vi "Grid_multiGridV3.vi"() -> ()   [LabVIEW 2014]
panel:
  out "size(s) 5":i32
  out "size(s) 4":i32
  out "size(s) 3":i32=11
  out "size(s) 2":i32=12
  out "size(s)":i32=15
  out "data\n\n 5":T1(array[cluster])=[{"Amplitude (mod. signal unit)"=0.0, "Lockin on/off status"=FALSE, "Backward sweep"=TRUE, "Number of points"=215, "Channels"=["Current (A)", "LI Demod 1 X (A)", "LI Demod 1 Y (A)", "LI Demod 2 X (A)", "LI Demod 2 Y (A)"], "Parameters"=["X (m)", "Y (m)", "Z (m)", "Z offset (m)", "Settling time (s)", "Integration time (s)", "Z-Ctrl hold", "Final Z (m)"], "Fixed parameters"=["Sweep Start", "Sweep End"], "Multiple sweeps configuration"={"Number of Sweeps"=1, "Save all"=FALSE}, "Initialization"={"Z averaging time (s)"=0.001, "Initial settling time (s)"=0.0002}, "Sweep Timing"={"Max. slew rate (V/s)"=inf, "Settling time (s)"=0.001, "Integration time (s)"=0.001}, "End of Sweep"={"End settling time (s)"=5e-05, "Z control time (s)"=0.0002}, "Initial Z-Offset (m)"=0.0, "Sweep Distance (m)"=0.0, "Channels 2"=[], "Name"="", "Reset Z"=FALSE, "Record final Z"=FALSE, "Auto Retract Status"=FALSE, "Threshold"=0.0, "Auto Retract Signal Index"=0, "Auto Retract Condition"=FALSE}, {"Amplitude (mod. signal unit)"=0.0, "Lockin on/off status"=FALSE, "Backward sweep"=FALSE, "Number of points"=0, "Channels"=[], "Parameters"=[], "Fixed parameters"=[], "Multiple sweeps configuration"={"Number of Sweeps"=0, "Save all"=FALSE}, "Initialization"={"Z averaging time (s)"=0.0, "Initial settling time (s)"=0.0}, "Sweep Timing"={"Max. slew rate (V/s)"=0.0, "Settling time (s)"=0.0, "Integration time (s)"=0.0}, "End of Sweep"={"End settling time (s)"=0.0, "Z control time (s)"=0.0}, "Initial Z-Offset (m)"=0.0, "Sweep Distance (m)"=0.0, "Channels 2"=[], "Name"="", "Reset Z"=FALSE, "Record final Z"=FALSE, "Auto Retract Status"=FALSE, "Threshold"=0.0, "Auto Retract Signal Index"=0, "Auto Retract Condition"=FALSE}, {"Amplitude (mod. signal unit)"=0.0, "Lockin on/off status"=FALSE, "Backward sweep"=FALSE, "Number of points"=0, "Channels"=[], "Parameters"=[], "Fixed parameters"=[], "Multiple sweeps configuration"={"Number of Sweeps"=0, "Save all"=FALSE}, "Initialization"={"Z averaging time (s)"=0.0, "Initial settling time (s)"=0.0}, "Sweep Timing"={"Max. slew rate (V/s)"=0.0, "Settling time (s)"=0.0, "Integration time (s)"=0.0}, "End of Sweep"={"End settling time (s)"=0.0, "Z control time (s)"=0.0}, "Initial Z-Offset (m)"=0.0, "Sweep Distance (m)"=0.0, "Channels 2"=[], "Name"="", "Reset Z"=FALSE, "Record final Z"=FALSE, "Auto Retract Status"=FALSE, "Threshold"=0.0, "Auto Retract Signal Index"=0, "Auto Retract Condition"=FALSE}, {"Amplitude (mod. signal unit)"=0.0, "Lockin on/off status"=FALSE, "Backward sweep"=FALSE, "Number of points"=0, "Channels"=[], "Parameters"=[], "Fixed parameters"=[], "Multiple sweeps configuration"={"Number of Sweeps"=0, "Save all"=FALSE}, "Initialization"={"Z averaging time (s)"=0.0, "Initial settling time (s)"=0.0}, "Sweep Timing"={"Max. slew rate (V/s)"=0.0, "Settling time (s)"=0.0, "Integration time (s)"=0.0}, "End of Sweep"={"End settling time (s)"=0.0, "Z control time (s)"=0.0}, "Initial Z-Offset (m)"=0.0, "Sweep Distance (m)"=0.0, "Channels 2"=[], "Name"="", "Reset Z"=FALSE, "Record final Z"=FALSE, "Auto Retract Status"=FALSE, "Threshold"=0.0, "Auto Retract Signal Index"=0, "Auto Retract Condition"=FALSE}, {"Amplitude (mod. signal unit)"=0.0, "Lockin on/off status"=FALSE, "Backward sweep"=FALSE, "Number of points"=0, "Channels"=[], "Parameters"=[], "Fixed parameters"=[], "Multiple sweeps configuration"={"Number of Sweeps"=0, "Save all"=FALSE}, "Initialization"={"Z averaging time (s)"=0.0, "Initial settling time (s)"=0.0}, "Sweep Timing"={"Max. slew rate (V/s)"=0.0, "Settling time (s)"=0.0, "Integration time (s)"=0.0}, "End of Sweep"={"End settling time (s)"=0.0, "Z control time (s)"=0.0}, "Initial Z-Offset (m)"=0.0, "Sweep Distance (m)"=0.0, "Channels 2"=[], "Name"="", "Reset Z"=FALSE, "Record final Z"=FALSE, "Auto Retract Status"=FALSE, "Threshold"=0.0, "Auto Retract Signal Index"=0, "Auto Retract Condition"=FALSE}, {"Amplitude (mod. signal unit)"=0.0, "Lockin on/off status"=FALSE, "Backward sweep"=FALSE, "Number of points"=0, "Channels"=[], "Parameters"=[], "Fixed parameters"=[], "Multiple sweeps configuration"={"Number of Sweeps"=0, "Save all"=FALSE}, "Initialization"={"Z averaging time (s)"=0.0, "Initial settling time (s)"=0.0}, "Sweep Timing"={"Max. slew rate (V/s)"=0.0, "Settling time (s)"=0.0, "Integration time (s)"=0.0}, "End of Sweep"={"End settling time (s)"=0.0, "Z control time (s)"=0.0}, "Initial Z-Offset (m)"=0.0, "Sweep Distance (m)"=0.0, "Channels 2"=[], "Name"="", "Reset Z"=FALSE, "Record final Z"=FALSE, "Auto Retract Status"=FALSE, "Threshold"=0.0, "Auto Retract Signal Index"=0, "Auto Retract Condition"=FALSE}, {"Amplitude (mod. signal unit)"=0.0, "Lockin on/off status"=FALSE, "Backward sweep"=FALSE, "Number of points"=0, "Channels"=[], "Parameters"=[], "Fixed parameters"=[], "Multiple sweeps configuration"={"Number of Sweeps"=0, "Save all"=FALSE}, "Initialization"={"Z averaging time (s)"=0.0, "Initial settling time (s)"=0.0}, "Sweep Timing"={"Max. slew rate (V/s)"=0.0, "Settling time (s)"=0.0, "Integration time (s)"=0.0}, "End of Sweep"={"End settling time (s)"=0.0, "Z control time (s)"=0.0}, "Initial Z-Offset (m)"=0.0, "Sweep Distance (m)"=0.0, "Channels 2"=[], "Name"="", "Reset Z"=FALSE, "Record final Z"=FALSE, "Auto Retract Status"=FALSE, "Threshold"=0.0, "Auto Retract Signal Index"=0, "Auto Retract Condition"=FALSE}, {"Amplitude (mod. signal unit)"=0.0, "Lockin on/off status"=FALSE, "Backward sweep"=FALSE, "Number of points"=0, "Channels"=[], "Parameters"=[], "Fixed parameters"=[], "Multiple sweeps configuration"={"Number of Sweeps"=0, "Save all"=FALSE}, "Initialization"={"Z averaging time (s)"=0.0, "Initial settling time (s)"=0.0}, "Sweep Timing"={"Max. slew rate (V/s)"=0.0, "Settling time (s)"=0.0, "Integration time (s)"=0.0}, "End of Sweep"={"End settling time (s)"=0.0, "Z control time (s)"=0.0}, "Initial Z-Offset (m)"=0.0, "Sweep Distance (m)"=0.0, "Channels 2"=[], "Name"="", "Reset Z"=FALSE, "Record final Z"=FALSE, "Auto Retract Status"=FALSE, "Threshold"=0.0, "Auto Retract Signal Index"=0, "Auto Retract Condition"=FALSE}, {"Amplitude (mod. signal unit)"=0.0, "Lockin on/off status"=FALSE, "Backward sweep"=FALSE, "Number of points"=0, "Channels"=[], "Parameters"=[], "Fixed parameters"=[], "Multiple sweeps configuration"={"Number of Sweeps"=0, "Save all"=FALSE}, "Initialization"={"Z averaging time (s)"=0.0, "Initial settling time (s)"=0.0}, "Sweep Timing"={"Max. slew rate (V/s)"=0.0, "Settling time (s)"=0.0, "Integration time (s)"=0.0}, "End of Sweep"={"End settling time (s)"=0.0, "Z control time (s)"=0.0}, "Initial Z-Offset (m)"=0.0, "Sweep Distance (m)"=0.0, "Channels 2"=[], "Name"="", "Reset Z"=FALSE, "Record final Z"=FALSE, "Auto Retract Status"=FALSE, "Threshold"=0.0, "Auto Retract Signal Index"=0, "Auto Retract Condition"=FALSE}, {"Amplitude (mod. signal unit)"=0.0, "Lockin on/off status"=FALSE, "Backward sweep"=FALSE, "Number of points"=0, "Channels"=[], "Parameters"=[], "Fixed parameters"=[], "Multiple sweeps configuration"={"Number of Sweeps"=0, "Save all"=FALSE}, "Initialization"={"Z averaging time (s)"=0.0, "Initial settling time (s)"=0.0}, "Sweep Timing"={"Max. slew rate (V/s)"=0.0, "Settling time (s)"=0.0, "Integration time (s)"=0.0}, "End of Sweep"={"End settling time (s)"=0.0, "Z control time (s)"=0.0}, "Initial Z-Offset (m)"=0.0, "Sweep Distance (m)"=0.0, "Channels 2"=[], "Name"="", "Reset Z"=FALSE, "Record final Z"=FALSE, "Auto Retract Status"=FALSE, "Threshold"=0.0, "Auto Retract Signal Index"=0, "Auto Retract Condition"=FALSE}, {"Amplitude (mod. signal unit)"=0.0, "Lockin on/off status"=FALSE, "Backward sweep"=FALSE, "Number of points"=0, "Channels"=[], "Parameters"=[], "Fixed parameters"=[], "Multiple sweeps configuration"={"Number of Sweeps"=0, "Save all"=FALSE}, "Initialization"={"Z averaging time (s)"=0.0, "Initial settling time (s)"=0.0}, "Sweep Timing"={"Max. slew rate (V/s)"=0.0, "Settling time (s)"=0.0, "Integration time (s)"=0.0}, "End of Sweep"={"End settling time (s)"=0.0, "Z control time (s)"=0.0}, "Initial Z-Offset (m)"=0.0, "Sweep Distance (m)"=0.0, "Channels 2"=[], "Name"="", "Reset Z"=FALSE, "Record final Z"=FALSE, "Auto Retract Status"=FALSE, "Threshold"=0.0, "Auto Retract Signal Index"=0, "Auto Retract Condition"=FALSE}, {"Amplitude (mod. signal unit)"=0.0, "Lockin on/off status"=FALSE, "Backward sweep"=FALSE, "Number of points"=0, "Channels"=[], "Parameters"=[], "Fixed parameters"=[], "Multiple sweeps configuration"={"Number of Sweeps"=0, "Save all"=FALSE}, "Initialization"={"Z averaging time (s)"=0.0, "Initial settling time (s)"=0.0}, "Sweep Timing"={"Max. slew rate (V/s)"=0.0, "Settling time (s)"=0.0, "Integration time (s)"=0.0}, "End of Sweep"={"End settling time (s)"=0.0, "Z control time (s)"=0.0}, "Initial Z-Offset (m)"=0.0, "Sweep Distance (m)"=0.0, "Channels 2"=[], "Name"="", "Reset Z"=FALSE, "Record final Z"=FALSE, "Auto Retract Status"=FALSE, "Threshold"=0.0, "Auto Retract Signal Index"=0, "Auto Retract Condition"=FALSE}, {"Amplitude (mod. signal unit)"=0.0, "Lockin on/off status"=FALSE, "Backward sweep"=FALSE, "Number of points"=0, "Channels"=[], "Parameters"=[], "Fixed parameters"=[], "Multiple sweeps configuration"={"Number of Sweeps"=0, "Save all"=FALSE}, "Initialization"={"Z averaging time (s)"=0.0, "Initial settling time (s)"=0.0}, "Sweep Timing"={"Max. slew rate (V/s)"=0.0, "Settling time (s)"=0.0, "Integration time (s)"=0.0}, "End of Sweep"={"End settling time (s)"=0.0, "Z control time (s)"=0.0}, "Initial Z-Offset (m)"=0.0, "Sweep Distance (m)"=0.0, "Channels 2"=[], "Name"="", "Reset Z"=FALSE, "Record final Z"=FALSE, "Auto Retract Status"=FALSE, "Threshold"=0.0, "Auto Retract Signal Index"=0, "Auto Retract Condition"=FALSE}, {"Amplitude (mod. signal unit)"=0.0, "Lockin on/off status"=FALSE, "Backward sweep"=FALSE, "Number of points"=0, "Channels"=[], "Parameters"=[], "Fixed parameters"=[], "Multiple sweeps configuration"={"Number of Sweeps"=0, "Save all"=FALSE}, "Initialization"={"Z averaging time (s)"=0.0, "Initial settling time (s)"=0.0}, "Sweep Timing"={"Max. slew rate (V/s)"=0.0, "Settling time (s)"=0.0, "Integration time (s)"=0.0}, "End of Sweep"={"End settling time (s)"=0.0, "Z control time (s)"=0.0}, "Initial Z-Offset (m)"=0.0, "Sweep Distance (m)"=0.0, "Channels 2"=[], "Name"="", "Reset Z"=FALSE, "Record final Z"=FALSE, "Auto Retract Status"=FALSE, "Threshold"=0.0, "Auto Retract Signal Index"=0, "Auto Retract Condition"=FALSE}, {"Amplitude (mod. signal unit)"=0.0, "Lockin on/off status"=FALSE, "Backward sweep"=FALSE, "Number of points"=0, "Channels"=[], "Parameters"=[], "Fixed parameters"=[], "Multiple sweeps configuration"={"Number of Sweeps"=0, "Save all"=FALSE}, "Initialization"={"Z averaging time (s)"=0.0, "Initial settling time (s)"=0.0}, "Sweep Timing"={"Max. slew rate (V/s)"=0.0, "Settling time (s)"=0.0, "Integration time (s)"=0.0}, "End of Sweep"={"End settling time (s)"=0.0, "Z control time (s)"=0.0}, "Initial Z-Offset (m)"=0.0, "Sweep Distance (m)"=0.0, "Channels 2"=[], "Name"="", "Reset Z"=FALSE, "Record final Z"=FALSE, "Auto Retract Status"=FALSE, "Threshold"=0.0, "Auto Retract Signal Index"=0, "Auto Retract Condition"=FALSE}, {"Amplitude (mod. signal unit)"=0.0, "Lockin on/off status"=FALSE, "Backward sweep"=FALSE, "Number of points"=0, "Channels"=[], "Parameters"=[], "Fixed parameters"=[], "Multiple sweeps configuration"={"Number of Sweeps"=0, "Save all"=FALSE}, "Initialization"={"Z averaging time (s)"=0.0, "Initial settling time (s)"=0.0}, "Sweep Timing"={"Max. slew rate (V/s)"=0.0, "Settling time (s)"=0.0, "Integration time (s)"=0.0}, "End of Sweep"={"End settling time (s)"=0.0, "Z control time (s)"=0.0}, "Initial Z-Offset (m)"=0.0, "Sweep Distance (m)"=0.0, "Channels 2"=[], "Name"="", "Reset Z"=FALSE, "Record final Z"=FALSE, "Auto Retract Status"=FALSE, "Threshold"=0.0, "Auto Retract Signal Index"=0, "Auto Retract Condition"=FALSE}, {"Amplitude (mod. signal unit)"=0.0, "Lockin on/off status"=FALSE, "Backward sweep"=FALSE, "Number of points"=0, "Channels"=[], "Parameters"=[], "Fixed parameters"=[], "Multiple sweeps configuration"={"Number of Sweeps"=0, "Save all"=FALSE}, "Initialization"={"Z averaging time (s)"=0.0, "Initial settling time (s)"=0.0}, "Sweep Timing"={"Max. slew rate (V/s)"=0.0, "Settling time (s)"=0.0, "Integration time (s)"=0.0}, "End of Sweep"={"End settling time (s)"=0.0, "Z control time (s)"=0.0}, "Initial Z-Offset (m)"=0.0, "Sweep Distance (m)"=0.0, "Channels 2"=[], "Name"="", "Reset Z"=FALSE, "Record final Z"=FALSE, "Auto Retract Status"=FALSE, "Threshold"=0.0, "Auto Retract Signal Index"=0, "Auto Retract Condition"=FALSE}, {"Amplitude (mod. signal unit)"=0.0, "Lockin on/off status"=FALSE, "Backward sweep"=FALSE, "Number of points"=0, "Channels"=[], "Parameters"=[], "Fixed parameters"=[], "Multiple sweeps configuration"={"Number of Sweeps"=0, "Save all"=FALSE}, "Initialization"={"Z averaging time (s)"=0.0, "Initial settling time (s)"=0.0}, "Sweep Timing"={"Max. slew rate (V/s)"=0.0, "Settling time (s)"=0.0, "Integration time (s)"=0.0}, "End of Sweep"={"End settling time (s)"=0.0, "Z control time (s)"=0.0}, "Initial Z-Offset (m)"=0.0, "Sweep Distance (m)"=0.0, "Channels 2"=[], "Name"="", "Reset Z"=FALSE, "Record final Z"=FALSE, "Auto Retract Status"=FALSE, "Threshold"=0.0, "Auto Retract Signal Index"=0, "Auto Retract Condition"=FALSE}]
  out "data\n\n 2":T2(array[cluster])=[{"Amplitude (mod. signal unit)"=0.0, "Lockin on/off status"=FALSE, "Advanced options"={"Z-Controller Hold"=TRUE, "Record final Z"=FALSE, "Reset Bias"=TRUE}, "Backward sweep"=TRUE, "Number of points"=215, "Channels"=["Current (A)", "LI Demod 1 X (A)", "LI Demod 1 Y (A)", "LI Demod 2 X (A)", "LI Demod 2 Y (A)"], "Parameters"=["X (m)", "Y (m)", "Z (m)", "Z offset (m)", "Settling time (s)", "Integration time (s)", "Z-Ctrl hold", "Final Z (m)"], "Fixed parameters"=["Sweep Start", "Sweep End"], "Multiple sweeps configuration"={"Number of Sweeps"=1, "Save all"=FALSE}, "Initialization"={"Z averaging time (s)"=0.001, "Z offset (m)"=0.0, "Initial settling time (s)"=0.0002}, "Sweep Timing"={"Max. slew rate (V/s)"=inf, "Settling time (s)"=0.001, "Integration time (s)"=0.001}, "End of Sweep"={"End settling time (s)"=5e-05, "Z control time (s)"=0.0002}, "Start value (V)"=-0.02, "End value (V)"=-3.0, "Channels 2"=[0, 20, 21, 22, 23], "Name"="numerical_DCA_-20mV->-3V"}, {"Amplitude (mod. signal unit)"=0.0, "Lockin on/off status"=FALSE, "Advanced options"={"Z-Controller Hold"=TRUE, "Record final Z"=FALSE, "Reset Bias"=TRUE}, "Backward sweep"=TRUE, "Number of points"=215, "Channels"=["Current (A)", "LI Demod 1 X (A)", "LI Demod 1 Y (A)", "LI Demod 2 X (A)", "LI Demod 2 Y (A)"], "Parameters"=["X (m)", "Y (m)", "Z (m)", "Z offset (m)", "Settling time (s)", "Integration time (s)", "Z-Ctrl hold", "Final Z (m)"], "Fixed parameters"=["Sweep Start", "Sweep End"], "Multiple sweeps configuration"={"Number of Sweeps"=1, "Save all"=FALSE}, "Initialization"={"Z averaging time (s)"=0.001, "Z offset (m)"=0.0, "Initial settling time (s)"=0.0002}, "Sweep Timing"={"Max. slew rate (V/s)"=inf, "Settling time (s)"=0.001, "Integration time (s)"=0.001}, "End of Sweep"={"End settling time (s)"=5e-05, "Z control time (s)"=0.0002}, "Start value (V)"=-0.02, "End value (V)"=0.7, "Channels 2"=[0, 20, 21, 22, 23], "Name"="numerical_DCA_-20mV->0.7V"}, {"Amplitude (mod. signal unit)"=0.0, "Lockin on/off status"=FALSE, "Advanced options"={"Z-Controller Hold"=TRUE, "Record final Z"=FALSE, "Reset Bias"=TRUE}, "Backward sweep"=TRUE, "Number of points"=215, "Channels"=["Current (A)", "LI Demod 1 X (A)", "LI Demod 1 Y (A)", "LI Demod 2 X (A)", "LI Demod 2 Y (A)"], "Parameters"=["X (m)", "Y (m)", "Z (m)", "Z offset (m)", "Settling time (s)", "Integration time (s)", "Z-Ctrl hold", "Final Z (m)"], "Fixed parameters"=["Sweep Start", "Sweep End"], "Multiple sweeps configuration"={"Number of Sweeps"=30, "Save all"=FALSE}, "Initialization"={"Z averaging time (s)"=0.001, "Z offset (m)"=0.0, "Initial settling time (s)"=0.0002}, "Sweep Timing"={"Max. slew rate (V/s)"=inf, "Settling time (s)"=0.001, "Integration time (s)"=0.001}, "End of Sweep"={"End settling time (s)"=5e-05, "Z control time (s)"=0.0002}, "Start value (V)"=-0.02, "End value (V)"=0.7, "Channels 2"=[0, 20, 21, 22, 23], "Name"="numerical_DCA_-20mV->-0.7V_30sweeps"}, {"Amplitude (mod. signal unit)"=0.0, "Lockin on/off status"=FALSE, "Advanced options"={"Z-Controller Hold"=TRUE, "Record final Z"=FALSE, "Reset Bias"=TRUE}, "Backward sweep"=TRUE, "Number of points"=215, "Channels"=["Current (A)", "LI Demod 1 X (A)", "LI Demod 1 Y (A)", "LI Demod 2 X (A)", "LI Demod 2 Y (A)"], "Parameters"=["X (m)", "Y (m)", "Z (m)", "Z offset (m)", "Settling time (s)", "Integration time (s)", "Z-Ctrl hold", "Final Z (m)"], "Fixed parameters"=["Sweep Start", "Sweep End"], "Multiple sweeps configuration"={"Number of Sweeps"=50, "Save all"=FALSE}, "Initialization"={"Z averaging time (s)"=0.001, "Z offset (m)"=0.0, "Initial settling time (s)"=0.0002}, "Sweep Timing"={"Max. slew rate (V/s)"=inf, "Settling time (s)"=0.001, "Integration time (s)"=0.001}, "End of Sweep"={"End settling time (s)"=5e-05, "Z control time (s)"=0.0002}, "Start value (V)"=-0.02, "End value (V)"=0.7, "Channels 2"=[0, 20, 21, 22, 23], "Name"="numerical_DCA_-20mV->-0.7V_50_sweeps"}, {"Amplitude (mod. signal unit)"=0.0, "Lockin on/off status"=FALSE, "Advanced options"={"Z-Controller Hold"=TRUE, "Record final Z"=FALSE, "Reset Bias"=TRUE}, "Backward sweep"=TRUE, "Number of points"=215, "Channels"=["Current (A)", "LI Demod 1 X (A)", "LI Demod 1 Y (A)", "LI Demod 2 X (A)", "LI Demod 2 Y (A)"], "Parameters"=["X (m)", "Y (m)", "Z (m)", "Z offset (m)", "Settling time (s)", "Integration time (s)", "Z-Ctrl hold", "Final Z (m)"], "Fixed parameters"=["Sweep Start", "Sweep End"], "Multiple sweeps configuration"={"Number of Sweeps"=70, "Save all"=FALSE}, "Initialization"={"Z averaging time (s)"=0.001, "Z offset (m)"=0.0, "Initial settling time (s)"=0.0002}, "Sweep Timing"={"Max. slew rate (V/s)"=inf, "Settling time (s)"=0.001, "Integration time (s)"=0.001}, "End of Sweep"={"End settling time (s)"=5e-05, "Z control time (s)"=0.0002}, "Start value (V)"=-0.02, "End value (V)"=-3.0, "Channels 2"=[0, 20, 21, 22, 23], "Name"="numerical_DCA_-20mV->-3V_70sweeps"}, {"Amplitude (mod. signal unit)"=0.0, "Lockin on/off status"=FALSE, "Advanced options"={"Z-Controller Hold"=TRUE, "Record final Z"=FALSE, "Reset Bias"=TRUE}, "Backward sweep"=TRUE, "Number of points"=215, "Channels"=["Current (A)", "LI Demod 1 X (A)", "LI Demod 1 Y (A)", "LI Demod 2 X (A)", "LI Demod 2 Y (A)"], "Parameters"=["X (m)", "Y (m)", "Z (m)", "Z offset (m)", "Settling time (s)", "Integration time (s)", "Z-Ctrl hold", "Final Z (m)"], "Fixed parameters"=["Sweep Start", "Sweep End"], "Multiple sweeps configuration"={"Number of Sweeps"=100, "Save all"=FALSE}, "Initialization"={"Z averaging time (s)"=0.001, "Z offset (m)"=0.0, "Initial settling time (s)"=0.0002}, "Sweep Timing"={"Max. slew rate (V/s)"=inf, "Settling time (s)"=0.001, "Integration time (s)"=0.001}, "End of Sweep"={"End settling time (s)"=5e-05, "Z control time (s)"=0.0002}, "Start value (V)"=-0.02, "End value (V)"=-3.0, "Channels 2"=[0, 20, 21, 22, 23], "Name"="numerical_DCA_-20mV->3V_100_sweeps"}, {"Amplitude (mod. signal unit)"=0.0, "Lockin on/off status"=FALSE, "Advanced options"={"Z-Controller Hold"=TRUE, "Record final Z"=FALSE, "Reset Bias"=TRUE}, "Backward sweep"=TRUE, "Number of points"=256, "Channels"=["Current (A)", "LI Demod 1 X (A)", "LI Demod 1 Y (A)", "LI Demod 2 X (A)", "LI Demod 2 Y (A)"], "Parameters"=["X (m)", "Y (m)", "Z (m)", "Z offset (m)", "Settling time (s)", "Integration time (s)", "Z-Ctrl hold", "Final Z (m)"], "Fixed parameters"=["Sweep Start", "Sweep End"], "Multiple sweeps configuration"={"Number of Sweeps"=100, "Save all"=FALSE}, "Initialization"={"Z averaging time (s)"=0.001, "Z offset (m)"=0.0, "Initial settling time (s)"=5e-05}, "Sweep Timing"={"Max. slew rate (V/s)"=inf, "Settling time (s)"=0.001, "Integration time (s)"=0.0005}, "End of Sweep"={"End settling time (s)"=5e-05, "Z control time (s)"=5e-05}, "Start value (V)"=-1.0, "End value (V)"=2.0, "Channels 2"=[0, 20, 21, 22, 23], "Name"="numerical_-1V->2V"}, {"Amplitude (mod. signal unit)"=0.0, "Lockin on/off status"=FALSE, "Advanced options"={"Z-Controller Hold"=TRUE, "Record final Z"=FALSE, "Reset Bias"=TRUE}, "Backward sweep"=TRUE, "Number of points"=256, "Channels"=["Current (A)", "LI Demod 1 X (A)", "LI Demod 1 Y (A)", "LI Demod 2 X (A)", "LI Demod 2 Y (A)"], "Parameters"=["X (m)", "Y (m)", "Z (m)", "Z offset (m)", "Settling time (s)", "Integration time (s)", "Z-Ctrl hold", "Final Z (m)"], "Fixed parameters"=["Sweep Start", "Sweep End"], "Multiple sweeps configuration"={"Number of Sweeps"=100, "Save all"=FALSE}, "Initialization"={"Z averaging time (s)"=0.001, "Z offset (m)"=0.0, "Initial settling time (s)"=5e-05}, "Sweep Timing"={"Max. slew rate (V/s)"=inf, "Settling time (s)"=0.001, "Integration time (s)"=0.0005}, "End of Sweep"={"End settling time (s)"=5e-05, "Z control time (s)"=5e-05}, "Start value (V)"=-0.02, "End value (V)"=0.02, "Channels 2"=[0, 20, 21, 22, 23], "Name"="numerical_-20mV->20mV"}, {"Amplitude (mod. signal unit)"=0.0, "Lockin on/off status"=FALSE, "Advanced options"={"Z-Controller Hold"=TRUE, "Record final Z"=FALSE, "Reset Bias"=TRUE}, "Backward sweep"=TRUE, "Number of points"=286, "Channels"=["Current (A)", "LI Demod 1 X (A)", "LI Demod 1 Y (A)", "LI Demod 2 X (A)", "LI Demod 2 Y (A)"], "Parameters"=["X (m)", "Y (m)", "Z (m)", "Z offset (m)", "Settling time (s)", "Integration time (s)", "Z-Ctrl hold", "Final Z (m)"], "Fixed parameters"=["Sweep Start", "Sweep End"], "Multiple sweeps configuration"={"Number of Sweeps"=50, "Save all"=FALSE}, "Initialization"={"Z averaging time (s)"=0.001, "Z offset (m)"=0.0, "Initial settling time (s)"=5e-05}, "Sweep Timing"={"Max. slew rate (V/s)"=inf, "Settling time (s)"=0.001, "Integration time (s)"=0.0005}, "End of Sweep"={"End settling time (s)"=5e-05, "Z control time (s)"=5e-05}, "Start value (V)"=-0.2, "End value (V)"=0.8, "Channels 2"=[0, 20, 21, 22, 23], "Name"="DCA_numerical_-0.2V->0.8V"}, {"Amplitude (mod. signal unit)"=0.0, "Lockin on/off status"=FALSE, "Advanced options"={"Z-Controller Hold"=TRUE, "Record final Z"=FALSE, "Reset Bias"=TRUE}, "Backward sweep"=TRUE, "Number of points"=421, "Channels"=["Current (A)", "LI Demod 1 X (A)", "LI Demod 1 Y (A)", "LI Demod 2 X (A)", "LI Demod 2 Y (A)"], "Parameters"=["X (m)", "Y (m)", "Z (m)", "Z offset (m)", "Settling time (s)", "Integration time (s)", "Z-Ctrl hold", "Final Z (m)"], "Fixed parameters"=["Sweep Start", "Sweep End"], "Multiple sweeps configuration"={"Number of Sweeps"=100, "Save all"=FALSE}, "Initialization"={"Z averaging time (s)"=0.001, "Z offset (m)"=0.0, "Initial settling time (s)"=5e-05}, "Sweep Timing"={"Max. slew rate (V/s)"=inf, "Settling time (s)"=0.001, "Integration time (s)"=0.0005}, "End of Sweep"={"End settling time (s)"=5e-05, "Z control time (s)"=5e-05}, "Start value (V)"=-2.0, "End value (V)"=2.2, "Channels 2"=[0, 20, 21, 22, 23], "Name"="numerical_-2V->2.2V"}, {"Amplitude (mod. signal unit)"=0.0, "Lockin on/off status"=FALSE, "Advanced options"={"Z-Controller Hold"=TRUE, "Record final Z"=FALSE, "Reset Bias"=TRUE}, "Backward sweep"=TRUE, "Number of points"=500, "Channels"=["Current (A)", "LI Demod 1 X (A)", "LI Demod 1 Y (A)", "LI Demod 2 X (A)", "LI Demod 2 Y (A)"], "Parameters"=["X (m)", "Y (m)", "Z (m)", "Z offset (m)", "Settling time (s)", "Integration time (s)", "Z-Ctrl hold", "Final Z (m)"], "Fixed parameters"=["Sweep Start", "Sweep End"], "Multiple sweeps configuration"={"Number of Sweeps"=20, "Save all"=FALSE}, "Initialization"={"Z averaging time (s)"=0.001, "Z offset (m)"=0.0, "Initial settling time (s)"=0.01}, "Sweep Timing"={"Max. slew rate (V/s)"=inf, "Settling time (s)"=0.001, "Integration time (s)"=0.001}, "End of Sweep"={"End settling time (s)"=0.1, "Z control time (s)"=0.001}, "Start value (V)"=-0.2, "End value (V)"=0.8, "Channels 2"=[0, 20, 21, 22, 23], "Name"="DCA_numerical2_-0.2V->0.8V"}, {"Amplitude (mod. signal unit)"=0.0015, "Lockin on/off status"=FALSE, "Advanced options"={"Z-Controller Hold"=TRUE, "Record final Z"=FALSE, "Reset Bias"=TRUE}, "Backward sweep"=TRUE, "Number of points"=80, "Channels"=["Current (A)", "LI Demod 1 X (A)", "LI Demod 1 Y (A)", "LI Demod 2 X (A)", "LI Demod 2 Y (A)"], "Parameters"=["X (m)", "Y (m)", "Z (m)", "Z offset (m)", "Settling time (s)", "Integration time (s)", "Z-Ctrl hold", "Final Z (m)"], "Fixed parameters"=["Sweep Start", "Sweep End"], "Multiple sweeps configuration"={"Number of Sweeps"=10, "Save all"=FALSE}, "Initialization"={"Z averaging time (s)"=0.001, "Z offset (m)"=0.0, "Initial settling time (s)"=0.0046}, "Sweep Timing"={"Max. slew rate (V/s)"=inf, "Settling time (s)"=0.0046, "Integration time (s)"=0.032}, "End of Sweep"={"End settling time (s)"=5e-05, "Z control time (s)"=5e-05}, "Start value (V)"=-0.02, "End value (V)"=0.02, "Channels 2"=[0, 20, 21, 22, 23], "Name"="lockin_-20mV->20mV"}, {"Amplitude (mod. signal unit)"=0.002, "Lockin on/off status"=FALSE, "Advanced options"={"Z-Controller Hold"=TRUE, "Record final Z"=FALSE, "Reset Bias"=TRUE}, "Backward sweep"=TRUE, "Number of points"=70, "Channels"=["Current (A)", "LI Demod 1 X (A)", "LI Demod 1 Y (A)", "LI Demod 2 X (A)", "LI Demod 2 Y (A)"], "Parameters"=["X (m)", "Y (m)", "Z (m)", "Z offset (m)", "Settling time (s)", "Integration time (s)", "Z-Ctrl hold", "Final Z (m)"], "Fixed parameters"=["Sweep Start", "Sweep End"], "Multiple sweeps configuration"={"Number of Sweeps"=10, "Save all"=FALSE}, "Initialization"={"Z averaging time (s)"=0.001, "Z offset (m)"=0.0, "Initial settling time (s)"=0.0046}, "Sweep Timing"={"Max. slew rate (V/s)"=inf, "Settling time (s)"=0.0046, "Integration time (s)"=0.032}, "End of Sweep"={"End settling time (s)"=5e-05, "Z control time (s)"=5e-05}, "Start value (V)"=-0.025, "End value (V)"=0.025, "Channels 2"=[0, 20, 21, 22, 23], "Name"="lockin_-25mV->25mV"}, {"Amplitude (mod. signal unit)"=0.002, "Lockin on/off status"=FALSE, "Advanced options"={"Z-Controller Hold"=TRUE, "Record final Z"=FALSE, "Reset Bias"=TRUE}, "Backward sweep"=TRUE, "Number of points"=70, "Channels"=["Current (A)", "LI Demod 1 X (A)", "LI Demod 1 Y (A)", "LI Demod 2 X (A)", "LI Demod 2 Y (A)"], "Parameters"=["X (m)", "Y (m)", "Z (m)", "Z offset (m)", "Settling time (s)", "Integration time (s)", "Z-Ctrl hold", "Final Z (m)"], "Fixed parameters"=["Sweep Start", "Sweep End"], "Multiple sweeps configuration"={"Number of Sweeps"=10, "Save all"=FALSE}, "Initialization"={"Z averaging time (s)"=0.001, "Z offset (m)"=0.0, "Initial settling time (s)"=0.0046}, "Sweep Timing"={"Max. slew rate (V/s)"=inf, "Settling time (s)"=0.0046, "Integration time (s)"=0.032}, "End of Sweep"={"End settling time (s)"=5e-05, "Z control time (s)"=5e-05}, "Start value (V)"=-0.025, "End value (V)"=0.025, "Channels 2"=[0, 20, 21, 22, 23], "Name"="test"}, {"Amplitude (mod. signal unit)"=0.0025, "Lockin on/off status"=FALSE, "Advanced options"={"Z-Controller Hold"=TRUE, "Record final Z"=FALSE, "Reset Bias"=TRUE}, "Backward sweep"=TRUE, "Number of points"=320, "Channels"=["Current (A)", "LI Demod 1 X (A)", "LI Demod 1 Y (A)", "LI Demod 2 X (A)", "LI Demod 2 Y (A)"], "Parameters"=["X (m)", "Y (m)", "Z (m)", "Z offset (m)", "Settling time (s)", "Integration time (s)", "Z-Ctrl hold", "Final Z (m)"], "Fixed parameters"=["Sweep Start", "Sweep End"], "Multiple sweeps configuration"={"Number of Sweeps"=1, "Save all"=FALSE}, "Initialization"={"Z averaging time (s)"=0.001, "Z offset (m)"=0.0, "Initial settling time (s)"=0.0046}, "Sweep Timing"={"Max. slew rate (V/s)"=inf, "Settling time (s)"=0.0046, "Integration time (s)"=0.0042}, "End of Sweep"={"End settling time (s)"=5e-05, "Z control time (s)"=5e-05}, "Start value (V)"=0.02, "End value (V)"=-0.02, "Channels 2"=[0, 20, 21, 22, 23], "Name"="lockin_highRes_20mV_-20mV"}, {"Amplitude (mod. signal unit)"=0.005, "Lockin on/off status"=FALSE, "Advanced options"={"Z-Controller Hold"=TRUE, "Record final Z"=FALSE, "Reset Bias"=TRUE}, "Backward sweep"=TRUE, "Number of points"=256, "Channels"=["Current (A)", "LI Demod 1 X (A)", "LI Demod 1 Y (A)", "LI Demod 2 X (A)", "LI Demod 2 Y (A)"], "Parameters"=["X (m)", "Y (m)", "Z (m)", "Z offset (m)", "Settling time (s)", "Integration time (s)", "Z-Ctrl hold", "Final Z (m)"], "Fixed parameters"=["Sweep Start", "Sweep End"], "Multiple sweeps configuration"={"Number of Sweeps"=2, "Save all"=FALSE}, "Initialization"={"Z averaging time (s)"=0.001, "Z offset (m)"=0.0, "Initial settling time (s)"=0.0033}, "Sweep Timing"={"Max. slew rate (V/s)"=inf, "Settling time (s)"=0.0033, "Integration time (s)"=0.0164}, "End of Sweep"={"End settling time (s)"=5e-05, "Z control time (s)"=5e-05}, "Start value (V)"=-1.0, "End value (V)"=2.0, "Channels 2"=[0, 20, 21, 22, 23], "Name"="lockin_slow"}, {"Amplitude (mod. signal unit)"=0.005, "Lockin on/off status"=FALSE, "Advanced options"={"Z-Controller Hold"=TRUE, "Record final Z"=FALSE, "Reset Bias"=TRUE}, "Backward sweep"=TRUE, "Number of points"=310, "Channels"=["Current (A)", "LI Demod 1 X (A)", "LI Demod 1 Y (A)", "LI Demod 2 X (A)", "LI Demod 2 Y (A)"], "Parameters"=["X (m)", "Y (m)", "Z (m)", "Z offset (m)", "Settling time (s)", "Integration time (s)", "Z-Ctrl hold", "Final Z (m)"], "Fixed parameters"=["Sweep Start", "Sweep End"], "Multiple sweeps configuration"={"Number of Sweeps"=2, "Save all"=FALSE}, "Initialization"={"Z averaging time (s)"=0.001, "Z offset (m)"=0.0, "Initial settling time (s)"=0.0031}, "Sweep Timing"={"Max. slew rate (V/s)"=inf, "Settling time (s)"=0.0031, "Integration time (s)"=0.0246}, "End of Sweep"={"End settling time (s)"=5e-05, "Z control time (s)"=5e-05}, "Start value (V)"=1.5, "End value (V)"=-0.05, "Channels 2"=[0, 20, 21, 22, 23], "Name"="Lock_in_DCA_1.5V->-50mV"}, {"Amplitude (mod. signal unit)"=0.005, "Lockin on/off status"=FALSE, "Advanced options"={"Z-Controller Hold"=TRUE, "Record final Z"=FALSE, "Reset Bias"=TRUE}, "Backward sweep"=TRUE, "Number of points"=401, "Channels"=["Current (A)", "Z (m)", "LI Demod 1 X (A)", "LI Demod 1 Y (A)", "LI Demod 2 X (A)", "LI Demod 2 Y (A)"], "Parameters"=["X (m)", "Y (m)", "Z (m)", "Z offset (m)", "Settling time (s)", "Integration time (s)", "Z-Ctrl hold", "Final Z (m)"], "Fixed parameters"=["Sweep Start", "Sweep End"], "Multiple sweeps configuration"={"Number of Sweeps"=1, "Save all"=FALSE}, "Initialization"={"Z averaging time (s)"=0.001, "Z offset (m)"=0.0, "Initial settling time (s)"=0.004}, "Sweep Timing"={"Max. slew rate (V/s)"=inf, "Settling time (s)"=0.02, "Integration time (s)"=0.015}, "End of Sweep"={"End settling time (s)"=5e-05, "Z control time (s)"=0.001}, "Start value (V)"=-1.0, "End value (V)"=1.0, "Channels 2"=[0, 14, 20, 21, 22, 23], "Name"="Long_MgPc_lockin_-1->1V"}, {"Amplitude (mod. signal unit)"=0.005, "Lockin on/off status"=FALSE, "Advanced options"={"Z-Controller Hold"=TRUE, "Record final Z"=FALSE, "Reset Bias"=TRUE}, "Backward sweep"=TRUE, "Number of points"=467, "Channels"=["Current (A)", "Z (m)", "LI Demod 1 X (A)", "LI Demod 1 Y (A)", "LI Demod 2 X (A)", "LI Demod 2 Y (A)"], "Parameters"=["X (m)", "Y (m)", "Z (m)", "Z offset (m)", "Settling time (s)", "Integration time (s)", "Z-Ctrl hold", "Final Z (m)"], "Fixed parameters"=["Sweep Start", "Sweep End"], "Multiple sweeps configuration"={"Number of Sweeps"=2, "Save all"=FALSE}, "Initialization"={"Z averaging time (s)"=0.001, "Z offset (m)"=0.0, "Initial settling time (s)"=0.004}, "Sweep Timing"={"Max. slew rate (V/s)"=inf, "Settling time (s)"=0.02, "Integration time (s)"=0.0246}, "End of Sweep"={"End settling time (s)"=5e-05, "Z control time (s)"=0.001}, "Start value (V)"=-2.0, "End value (V)"=1.5, "Channels 2"=[0, 14, 20, 21, 22, 23], "Name"="MgPc_long_lockin"}, {"Amplitude (mod. signal unit)"=0.008, "Lockin on/off status"=FALSE, "Advanced options"={"Z-Controller Hold"=TRUE, "Record final Z"=FALSE, "Reset Bias"=TRUE}, "Backward sweep"=TRUE, "Number of points"=256, "Channels"=["Current (A)", "LI Demod 1 X (A)", "LI Demod 1 Y (A)", "LI Demod 2 X (A)", "LI Demod 2 Y (A)"], "Parameters"=["X (m)", "Y (m)", "Z (m)", "Z offset (m)", "Settling time (s)", "Integration time (s)", "Z-Ctrl hold", "Final Z (m)"], "Fixed parameters"=["Sweep Start", "Sweep End"], "Multiple sweeps configuration"={"Number of Sweeps"=3, "Save all"=FALSE}, "Initialization"={"Z averaging time (s)"=0.001, "Z offset (m)"=0.0, "Initial settling time (s)"=0.0033}, "Sweep Timing"={"Max. slew rate (V/s)"=inf, "Settling time (s)"=0.0033, "Integration time (s)"=0.0082}, "End of Sweep"={"End settling time (s)"=5e-05, "Z control time (s)"=5e-05}, "Start value (V)"=-1.0, "End value (V)"=2.0, "Channels 2"=[0, 20, 21, 22, 23], "Name"="lockin_slow_-1_2"}, {"Amplitude (mod. signal unit)"=0.008, "Lockin on/off status"=FALSE, "Advanced options"={"Z-Controller Hold"=TRUE, "Record final Z"=FALSE, "Reset Bias"=TRUE}, "Backward sweep"=TRUE, "Number of points"=421, "Channels"=["Current (A)", "Z (m)", "LI Demod 1 X (A)", "LI Demod 1 Y (A)", "LI Demod 2 X (A)", "LI Demod 2 Y (A)"], "Parameters"=["X (m)", "Y (m)", "Z (m)", "Z offset (m)", "Settling time (s)", "Integration time (s)", "Z-Ctrl hold", "Final Z (m)"], "Fixed parameters"=["Sweep Start", "Sweep End"], "Multiple sweeps configuration"={"Number of Sweeps"=2, "Save all"=FALSE}, "Initialization"={"Z averaging time (s)"=0.001, "Z offset (m)"=0.0, "Initial settling time (s)"=5e-05}, "Sweep Timing"={"Max. slew rate (V/s)"=inf, "Settling time (s)"=0.0164, "Integration time (s)"=0.0164}, "End of Sweep"={"End settling time (s)"=5e-05, "Z control time (s)"=0.001}, "Start value (V)"=-2.0, "End value (V)"=2.2, "Channels 2"=[0, 14, 20, 21, 22, 23], "Name"="MgPc_long_lockin2"}, {"Amplitude (mod. signal unit)"=0.01, "Lockin on/off status"=FALSE, "Advanced options"={"Z-Controller Hold"=TRUE, "Record final Z"=FALSE, "Reset Bias"=TRUE}, "Backward sweep"=TRUE, "Number of points"=512, "Channels"=["Current (A)", "LI Demod 1 X (A)", "LI Demod 1 Y (A)", "LI Demod 2 X (A)", "LI Demod 2 Y (A)"], "Parameters"=["X (m)", "Y (m)", "Z (m)", "Z offset (m)", "Settling time (s)", "Integration time (s)", "Z-Ctrl hold", "Final Z (m)"], "Fixed parameters"=["Sweep Start", "Sweep End"], "Multiple sweeps configuration"={"Number of Sweeps"=1, "Save all"=FALSE}, "Initialization"={"Z averaging time (s)"=0.001, "Z offset (m)"=0.0, "Initial settling time (s)"=0.2}, "Sweep Timing"={"Max. slew rate (V/s)"=inf, "Settling time (s)"=0.0082, "Integration time (s)"=0.041}, "End of Sweep"={"End settling time (s)"=5e-05, "Z control time (s)"=5e-05}, "Start value (V)"=-3.0, "End value (V)"=2.0, "Channels 2"=[0, 20, 21, 22, 23], "Name"="Quick_Lockin"}]
  in  "Save As":string
  in  "Zspecparam.txt location":path=path "D:/Scripts/STSparam - Copy (2).txt"
  in  "Save As 2":string
  in  "STSparam.txt location":path=path "D:/Scripts/STSparam.txt"
  in  "Update STS/Zspec Param List":bool
  in  "START EXPERIMENT":bool
  in  "stop":bool
  in  "Duplicate Page 1":bool
  in  "No. of Exp":dbl=4.0 caption="No. of Experiments \n(If more than 5, edit VI)" step=1.0
  in  "Tab Control":T3(tab)=enum."Page 3"
  in  "Experiment 1":T4={"Drift Correction Settings"={"Drift Correction every"=6, "Drift correction Pixels"=128, "Channel index (0-23)"=0, "MaxImagesBack"=2, "Threshold"=2, "Increment"=1, "max applied Drift Correction"=40, "Correct Drift"=TRUE, "Correlate"=0, "Correct z drift"=FALSE, "zdrift \nDuration (s)"=0.0}, "Spectroscopy Setting"={"Imaging Current"=5e-11, "ref Current"=5e-12, "tip Speed (m/s)"=1e-08, "Imaging Bias"=-2.4, "ref Bias"=-0.02, "preSTS delay [ms]"=500, "STS z offset"=1e-11, "during Spec Bias (V)"=-0.02, "trigger1 < Hz"=0.0, "trigger 2 >Hz"=0.0, "autoStop"=FALSE, "Spectroscopy"=0, "PLL ON/OFF"=FALSE, "readjust setpoint every "=1, "z Reference"=TRUE, "Lock In"=FALSE}, "Misc"={"File name"="DCA_Zdependence_STS_Pos_Bias_Mol5_1_zOffset=10pm", "Email when finished"="Dhaneesh.Gopalakrishnan@monash.edu"}, "Grid Settings"={"type"=0, "type order"=0, "X pixel"=11, "Y pixel"=1, "Grid_Parms"={"center X (m)"=0.0, "center Y (m)"=0.0, "width (m)"=0.0, "height (m)"=0.0, "angle (deg)"=0.0}}, "STS Param List #1 "=3, "ZSpec Param List #1  "=0, "Repeat Experiment"={"Repeat"=TRUE, "Repeat Parameter"=2, "Values List #1"=7}} {"Repeat Experiment"."Repeat Parameter" items=["ref Current", "ref Bias", "STS z offset", "during Spec Bias (V)"]; "STS Param List #1" items=["numerical_DCA_-20mV->-3V", "numerical_DCA_-20mV->0.7V", "numerical_DCA_-20mV->-0.7V_30sweeps", "numerical_DCA_-20mV->-0.7V_50_sweeps", "numerical_DCA_-20mV->-3V_70sweeps", "numerical_DCA_-20mV->3V_100_sweeps", "numerical_-1V->2V", "numerical_-20mV->20mV", "DCA_numerical_-0.2V->0.8V", "numerical_-2V->2.2V", "DCA_numerical2_-0.2V->0.8V", "lockin_-20mV->20mV", "lockin_-25mV->25mV", "test", "lockin_highRes_20mV_-20mV", "lockin_slow", "Lock_in_DCA_1.5V->-50mV", "Long_MgPc_lockin_-1->1V", "MgPc_long_lockin", "lockin_slow_-1_2", "MgPc_long_lockin2", "Quick_Lockin"]; "Grid Settings"."type order" items=["Grid", "Random", "Adam7"]; "Grid Settings"."type" items=["Line", "Grid"]; "Spectroscopy Setting"."Spectroscopy" items=["Bias", "zSpec"]; "Spectroscopy Setting"."trigger 2 >Hz" format="%#_6p"; "Spectroscopy Setting"."trigger1 < Hz" format="%#_6p"; "Spectroscopy Setting"."during Spec Bias (V)" format="%#_5p"; "Spectroscopy Setting"."STS z offset" format="%#_6p"; "Spectroscopy Setting"."ref Bias" format="%#_6p"; "Spectroscopy Setting"."Imaging Bias" format="%#_6p"; "Spectroscopy Setting"."tip Speed (m/s)" format="%.2p"; "Spectroscopy Setting"."ref Current" format="%#_6p"; "Spectroscopy Setting"."Imaging Current" format="%#_6p"; "Drift Correction Settings"."Correlate" items=["first Frame", "successive Frames"]; "Drift Correction Settings"."max applied Drift Correction" min=1 max=100 step=1 format="%.0p"; "Drift Correction Settings"."Threshold" min=1 step=1; "Drift Correction Settings"."Channel index (0-23)" items=["Current"=0, "Z (m)"=14]}
  in  "Experiment 2":T5={"Drift Correction Settings"={"Drift Correction every"=6, "Drift correction Pixels"=128, "Channel index (0-23)"=0, "MaxImagesBack"=2, "Threshold"=2, "Increment"=1, "max applied Drift Correction"=40, "Correct Drift"=TRUE, "Correlate"=0, "Correct z drift"=FALSE, "zdrift \nDuration (s)"=0.0}, "Spectroscopy Setting"={"Imaging Current"=5e-11, "ref Current"=5e-12, "tip Speed (m/s)"=1e-08, "Imaging Bias"=-2.4, "ref Bias"=-0.02, "preSTS delay [ms]"=500, "STS z offset"=-1.1e-10, "during Spec Bias (V)"=-0.02, "trigger1 < Hz"=0.0, "trigger 2 >Hz"=0.0, "autoStop"=FALSE, "Spectroscopy"=0, "PLL ON/OFF"=FALSE, "readjust setpoint every "=1, "z Reference"=TRUE, "Lock In"=FALSE}, "Misc"={"File name"="DCA_Zdependence_STS_Pos_Bias_Mol5_1_zOffset=-110pm", "Email when finished"="Dhaneesh.Gopalakrishnan@monash.edu"}, "Grid Settings"={"type"=0, "type order"=0, "X pixel"=11, "Y pixel"=1, "Grid_Parms"={"center X (m)"=0.0, "center Y (m)"=0.0, "width (m)"=0.0, "height (m)"=0.0, "angle (deg)"=0.0}}, "STS Param List #2 "=2, "ZSpec Param List  #2 "=0, "Repeat Experiment"={"Repeat"=TRUE, "Repeat Parameter"=2, "Values List #2"=7}} {"Repeat Experiment"."Repeat Parameter" items=["ref Current", "ref Bias", "STS z offset", "during Spec Bias (V)"]; "STS Param List #2" items=["numerical_DCA_-20mV->-3V", "numerical_DCA_-20mV->0.7V", "numerical_DCA_-20mV->-0.7V_30sweeps", "numerical_DCA_-20mV->-0.7V_50_sweeps", "numerical_DCA_-20mV->-3V_70sweeps", "numerical_DCA_-20mV->3V_100_sweeps", "numerical_-1V->2V", "numerical_-20mV->20mV", "DCA_numerical_-0.2V->0.8V", "numerical_-2V->2.2V", "DCA_numerical2_-0.2V->0.8V", "lockin_-20mV->20mV", "lockin_-25mV->25mV", "test", "lockin_highRes_20mV_-20mV", "lockin_slow", "Lock_in_DCA_1.5V->-50mV", "Long_MgPc_lockin_-1->1V", "MgPc_long_lockin", "lockin_slow_-1_2", "MgPc_long_lockin2", "Quick_Lockin"]; "Grid Settings"."type order" items=["Grid", "Random", "Adam7"]; "Grid Settings"."type" items=["Line", "Grid"]; "Spectroscopy Setting"."Spectroscopy" items=["Bias", "zSpec"]; "Spectroscopy Setting"."trigger 2 >Hz" format="%#_6p"; "Spectroscopy Setting"."trigger1 < Hz" format="%#_6p"; "Spectroscopy Setting"."during Spec Bias (V)" format="%#_5p"; "Spectroscopy Setting"."STS z offset" format="%#_6p"; "Spectroscopy Setting"."ref Bias" format="%#_6p"; "Spectroscopy Setting"."Imaging Bias" format="%#_6p"; "Spectroscopy Setting"."tip Speed (m/s)" format="%.2p"; "Spectroscopy Setting"."ref Current" format="%#_6p"; "Spectroscopy Setting"."Imaging Current" format="%#_6p"; "Drift Correction Settings"."Correlate" items=["first Frame", "successive Frames"]; "Drift Correction Settings"."max applied Drift Correction" min=1 max=100 step=1 format="%.0p"; "Drift Correction Settings"."Threshold" min=1 step=1; "Drift Correction Settings"."Channel index (0-23)" items=["Current"=0, "Z (m)"=14]}
  in  "Experiment 3":T6={"Drift Correction Settings"={"Drift Correction every"=6, "Drift correction Pixels"=128, "Channel index (0-23)"=0, "MaxImagesBack"=2, "Threshold"=2, "Increment"=1, "max applied Drift Correction"=40, "Correct Drift"=TRUE, "Correlate"=0, "Correct z drift"=FALSE, "zdrift \nDuration (s)"=0.0}, "Spectroscopy Setting"={"Imaging Current"=5e-11, "ref Current"=5e-12, "tip Speed (m/s)"=1e-08, "Imaging Bias"=-2.4, "ref Bias"=-0.02, "preSTS delay [ms]"=500, "STS z offset"=4e-10, "during Spec Bias (V)"=-0.02, "trigger1 < Hz"=0.0, "trigger 2 >Hz"=0.0, "autoStop"=FALSE, "Spectroscopy"=0, "PLL ON/OFF"=FALSE, "readjust setpoint every "=1, "z Reference"=TRUE, "Lock In"=FALSE}, "Misc"={"File name"="DCA_Zdependence_STS_Neg_Bias_Mol5_1", "Email when finished"="Dhaneesh.Gopalakrishnan@monash.edu"}, "Grid Settings"={"type"=0, "type order"=0, "X pixel"=6, "Y pixel"=1, "Grid_Parms"={"center X (m)"=0.0, "center Y (m)"=0.0, "width (m)"=0.0, "height (m)"=0.0, "angle (deg)"=0.0}}, "STS Param List #3 "=4, "ZSpec Param List #3 "=0, "Repeat Experiment"={"Repeat"=TRUE, "Repeat Parameter"=2, "Values List #3"=7}} {"Repeat Experiment"."Repeat Parameter" items=["ref Current", "ref Bias", "STS z offset", "during Spec Bias (V)"]; "STS Param List #3" items=["numerical_DCA_-20mV->-3V", "numerical_DCA_-20mV->0.7V", "numerical_DCA_-20mV->-0.7V_30sweeps", "numerical_DCA_-20mV->-0.7V_50_sweeps", "numerical_DCA_-20mV->-3V_70sweeps", "numerical_DCA_-20mV->3V_100_sweeps", "numerical_-1V->2V", "numerical_-20mV->20mV", "DCA_numerical_-0.2V->0.8V", "numerical_-2V->2.2V", "DCA_numerical2_-0.2V->0.8V", "lockin_-20mV->20mV", "lockin_-25mV->25mV", "test", "lockin_highRes_20mV_-20mV", "lockin_slow", "Lock_in_DCA_1.5V->-50mV", "Long_MgPc_lockin_-1->1V", "MgPc_long_lockin", "lockin_slow_-1_2", "MgPc_long_lockin2", "Quick_Lockin"]; "Grid Settings"."type order" items=["Grid", "Random", "Adam7"]; "Grid Settings"."type" items=["Line", "Grid"]; "Spectroscopy Setting"."Spectroscopy" items=["Bias", "zSpec"]; "Spectroscopy Setting"."trigger 2 >Hz" format="%#_6p"; "Spectroscopy Setting"."trigger1 < Hz" format="%#_6p"; "Spectroscopy Setting"."during Spec Bias (V)" format="%#_5p"; "Spectroscopy Setting"."STS z offset" format="%#_6p"; "Spectroscopy Setting"."ref Bias" format="%#_6p"; "Spectroscopy Setting"."Imaging Bias" format="%#_6p"; "Spectroscopy Setting"."tip Speed (m/s)" format="%.2p"; "Spectroscopy Setting"."ref Current" format="%#_6p"; "Spectroscopy Setting"."Imaging Current" format="%#_6p"; "Drift Correction Settings"."Correlate" items=["first Frame", "successive Frames"]; "Drift Correction Settings"."max applied Drift Correction" min=1 max=100 step=1 format="%.0p"; "Drift Correction Settings"."Threshold" min=1 step=1; "Drift Correction Settings"."Channel index (0-23)" items=["Current"=0, "Z (m)"=14]}
  in  "Experiment 4":T7={"Drift Correction Settings"={"Drift Correction every"=1, "Drift correction Pixels"=128, "Channel index (0-23)"=0, "MaxImagesBack"=2, "Threshold"=2, "Increment"=1, "max applied Drift Correction"=40, "Correct Drift"=TRUE, "Correlate"=0, "Correct z drift"=FALSE, "zdrift \nDuration (s)"=0.0}, "Spectroscopy Setting"={"Imaging Current"=5e-11, "ref Current"=5e-12, "tip Speed (m/s)"=1e-08, "Imaging Bias"=-2.4, "ref Bias"=-0.02, "preSTS delay [ms]"=500, "STS z offset"=0.0, "during Spec Bias (V)"=-0.02, "trigger1 < Hz"=0.0, "trigger 2 >Hz"=0.0, "autoStop"=FALSE, "Spectroscopy"=0, "PLL ON/OFF"=FALSE, "readjust setpoint every "=1, "z Reference"=TRUE, "Lock In"=FALSE}, "Misc"={"File name"="DCA_Zdependence_STS_Neg_Bias_Mol5_1", "Email when finished"="Dhaneesh.Gopalakrishnan@monash.edu"}, "Grid Settings"={"type"=0, "type order"=0, "X pixel"=6, "Y pixel"=1, "Grid_Parms"={"center X (m)"=0.0, "center Y (m)"=0.0, "width (m)"=0.0, "height (m)"=0.0, "angle (deg)"=0.0}}, "STS Param List #4 "=0, "ZSpec Param List  #4"=0, "Repeat Experiment"={"Repeat"=TRUE, "Repeat Parameter"=2, "Values List #4"=7}} {"Repeat Experiment"."Repeat Parameter" items=["ref Current", "ref Bias", "STS z offset", "during Spec Bias (V)"]; "STS Param List #4" items=["numerical_DCA_-20mV->-3V", "numerical_DCA_-20mV->0.7V", "numerical_DCA_-20mV->-0.7V_30sweeps", "numerical_DCA_-20mV->-0.7V_50_sweeps", "numerical_DCA_-20mV->-3V_70sweeps", "numerical_DCA_-20mV->3V_100_sweeps", "numerical_-1V->2V", "numerical_-20mV->20mV", "DCA_numerical_-0.2V->0.8V", "numerical_-2V->2.2V", "DCA_numerical2_-0.2V->0.8V", "lockin_-20mV->20mV", "lockin_-25mV->25mV", "test", "lockin_highRes_20mV_-20mV", "lockin_slow", "Lock_in_DCA_1.5V->-50mV", "Long_MgPc_lockin_-1->1V", "MgPc_long_lockin", "lockin_slow_-1_2", "MgPc_long_lockin2", "Quick_Lockin"]; "Grid Settings"."type order" items=["Grid", "Random", "Adam7"]; "Grid Settings"."type" items=["Line", "Grid"]; "Spectroscopy Setting"."Spectroscopy" items=["Bias", "zSpec"]; "Spectroscopy Setting"."trigger 2 >Hz" format="%#_6p"; "Spectroscopy Setting"."trigger1 < Hz" format="%#_6p"; "Spectroscopy Setting"."during Spec Bias (V)" format="%#_5p"; "Spectroscopy Setting"."STS z offset" format="%#_6p"; "Spectroscopy Setting"."ref Bias" format="%#_6p"; "Spectroscopy Setting"."Imaging Bias" format="%#_6p"; "Spectroscopy Setting"."tip Speed (m/s)" format="%.2p"; "Spectroscopy Setting"."ref Current" format="%#_6p"; "Spectroscopy Setting"."Imaging Current" format="%#_6p"; "Drift Correction Settings"."Correlate" items=["first Frame", "successive Frames"]; "Drift Correction Settings"."max applied Drift Correction" min=1 max=100 step=1 format="%.0p"; "Drift Correction Settings"."Threshold" min=1 step=1; "Drift Correction Settings"."Channel index (0-23)" items=["Current"=0, "Z (m)"=14]}
  in  "Experiment 5":T8={"Drift Correction Settings"={"Drift Correction every"=1, "Drift correction Pixels"=256, "Channel index (0-23)"=0, "MaxImagesBack"=2, "Threshold"=2, "Increment"=1, "max applied Drift Correction"=40, "Correct Drift"=TRUE, "Correlate"=0, "Correct z drift"=FALSE, "zdrift \nDuration (s)"=0.0}, "Spectroscopy Setting"={"Imaging Current"=5e-11, "ref Current"=5e-12, "tip Speed (m/s)"=1e-08, "Imaging Bias"=-2.4, "ref Bias"=-0.02, "preSTS delay [ms]"=500, "STS z offset"=0.0, "during Spec Bias (V)"=-0.02, "trigger1 < Hz"=0.0, "trigger 2 >Hz"=0.0, "autoStop"=FALSE, "Spectroscopy"=0, "PLL ON/OFF"=FALSE, "readjust setpoint every "=1, "z Reference"=TRUE, "Lock In"=FALSE}, "Misc"={"File name"="DCA_Zdependence_STS_Pos_Bias_Mol9_46", "Email when finished"="Dhaneesh.Gopalakrishnan@monash.edu"}, "Grid Settings"={"type"=0, "type order"=0, "X pixel"=27, "Y pixel"=1, "Grid_Parms"={"center X (m)"=0.0, "center Y (m)"=0.0, "width (m)"=0.0, "height (m)"=0.0, "angle (deg)"=0.0}}, "STS Param List #5 "=0, "ZSpec Param List #5  "=0, "Repeat Experiment"={"Repeat"=TRUE, "Repeat Parameter"=2, "Values List #5"=7}} {"Repeat Experiment"."Repeat Parameter" items=["ref Current", "ref Bias", "STS z offset", "during Spec Bias (V)"]; "STS Param List #5" items=["numerical_DCA_-20mV->-3V", "numerical_DCA_-20mV->0.7V", "numerical_DCA_-20mV->-0.7V_30sweeps", "numerical_DCA_-20mV->-0.7V_50_sweeps", "numerical_DCA_-20mV->-3V_70sweeps", "numerical_DCA_-20mV->3V_100_sweeps", "numerical_-1V->2V", "numerical_-20mV->20mV", "DCA_numerical_-0.2V->0.8V", "numerical_-2V->2.2V", "DCA_numerical2_-0.2V->0.8V", "lockin_-20mV->20mV", "lockin_-25mV->25mV", "test", "lockin_highRes_20mV_-20mV", "lockin_slow", "Lock_in_DCA_1.5V->-50mV", "Long_MgPc_lockin_-1->1V", "MgPc_long_lockin", "lockin_slow_-1_2", "MgPc_long_lockin2", "Quick_Lockin"]; "Grid Settings"."type order" items=["Grid", "Random", "Adam7"]; "Grid Settings"."type" items=["Line", "Grid"]; "Spectroscopy Setting"."Spectroscopy" items=["Bias", "zSpec"]; "Spectroscopy Setting"."trigger 2 >Hz" format="%#_6p"; "Spectroscopy Setting"."trigger1 < Hz" format="%#_6p"; "Spectroscopy Setting"."during Spec Bias (V)" format="%#_5p"; "Spectroscopy Setting"."STS z offset" format="%#_6p"; "Spectroscopy Setting"."ref Bias" format="%#_6p"; "Spectroscopy Setting"."Imaging Bias" format="%#_6p"; "Spectroscopy Setting"."tip Speed (m/s)" format="%.2p"; "Spectroscopy Setting"."ref Current" format="%#_6p"; "Spectroscopy Setting"."Imaging Current" format="%#_6p"; "Drift Correction Settings"."Correlate" items=["first Frame", "successive Frames"]; "Drift Correction Settings"."max applied Drift Correction" min=1 max=100 step=1 format="%.0p"; "Drift Correction Settings"."Threshold" min=1 step=1; "Drift Correction Settings"."Channel index (0-23)" items=["Current"=0, "Z (m)"=14]}
  # "z Spectroscopy"
  # "GRID points"
  # "Increase this if no Drift was detected for \na certain number of images"
  # "% of image size"
  # "Only first frame works"
  # "z Spectroscopy"
  # "GRID points"
  # "Increase this if no Drift was detected for \na certain number of images"
  # "% of image size"
  # "Only first frame works"
  # "z Spectroscopy"
  # "GRID points"
  # "Increase this if no Drift was detected for \na certain number of images"
  # "% of image size"
  # "Only first frame works"
  # "z Spectroscopy"
  # "GRID points"
  # "Increase this if no Drift was detected for \na certain number of images"
  # "% of image size"
  # "Only first frame works"
  # "z Spectroscopy"
  # "GRID points"
  # "Increase this if no Drift was detected for \na certain number of images"
  # "% of image size"
  # "Only first frame works"
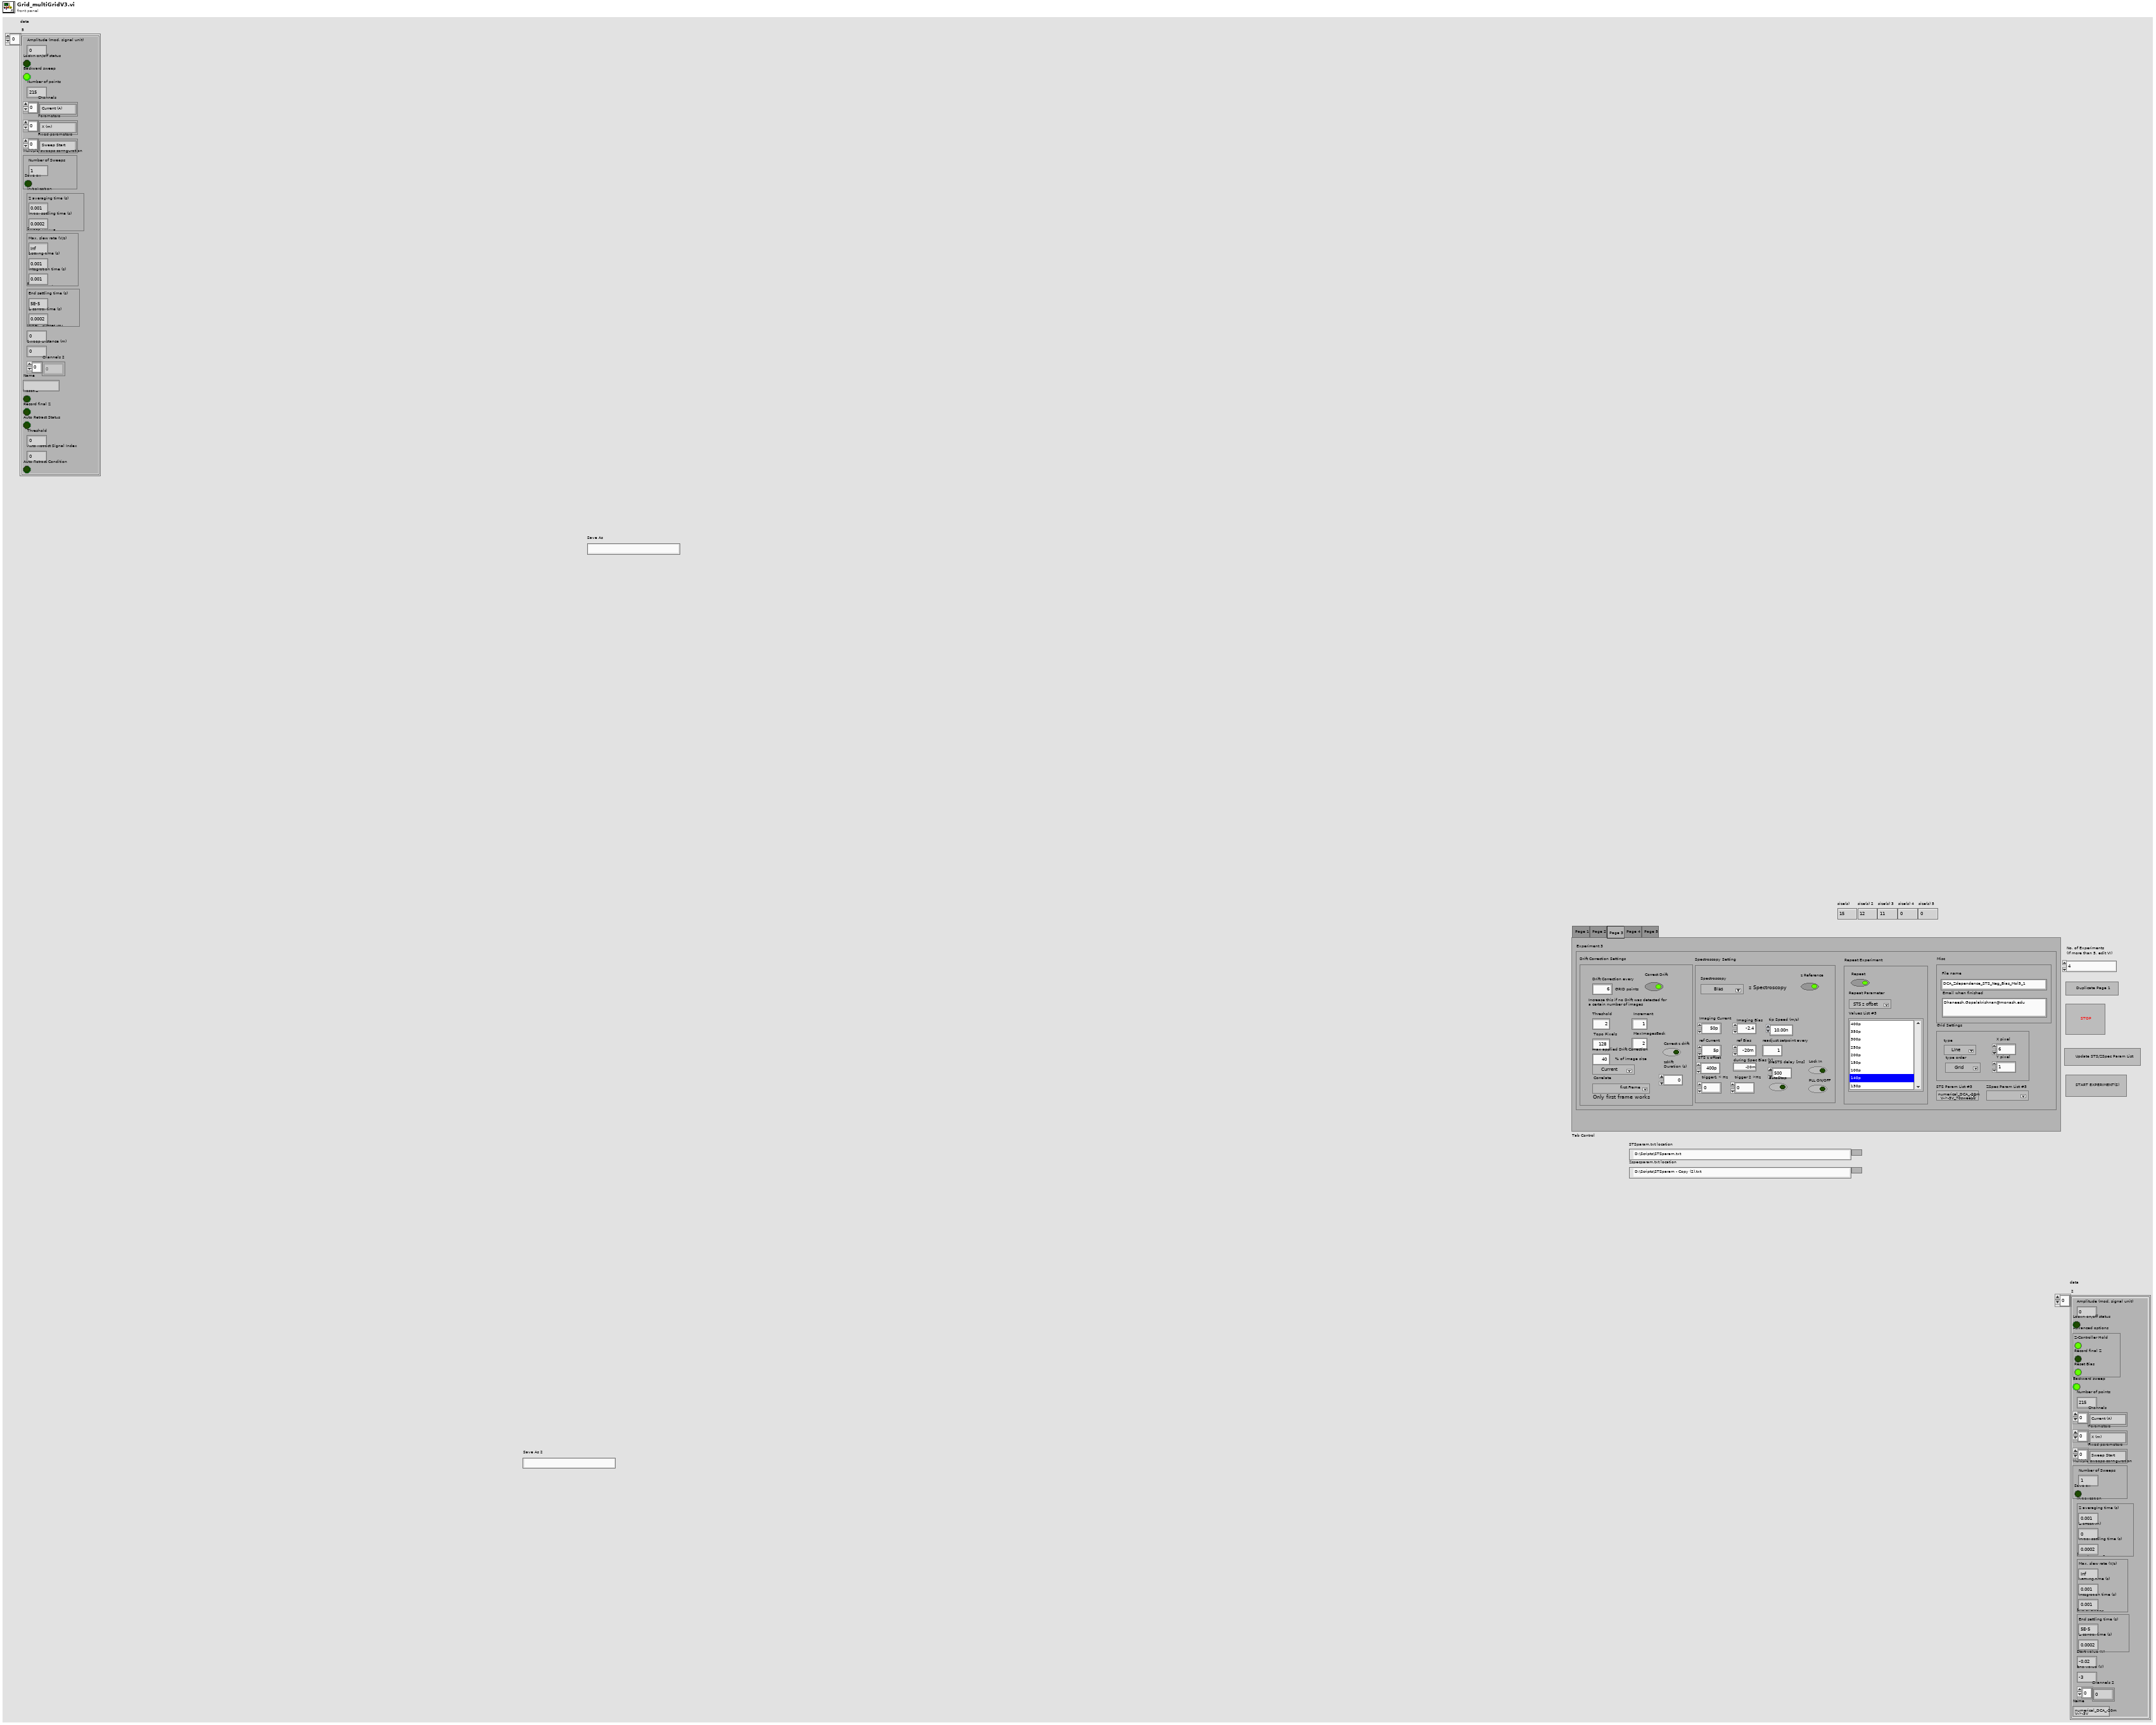
[diagram p1: front panel]
types:
  T1 = cluster{"Amplitude (mod. signal unit)":sgl, "Lockin on/off status":bool, "Backward sweep":bool, "Number of points":i32, "Channels":string[], "Parameters":string[], "Fixed parameters":string[], "Multiple sweeps configuration":cluster{"Number of Sweeps":i32, "Save all":bool}, "Initialization":cluster{"Z averaging time (s)":sgl, "Initial settling time (s)":sgl}, "Sweep Timing":cluster{"Max. slew rate (V/s)":sgl, "Settling time (s)":sgl, "Integration time (s)":sgl}, "End of Sweep":cluster{"End settling time (s)":sgl, "Z control time (s)":sgl}, "Initial Z-Offset (m)":sgl, "Sweep Distance (m)":sgl, "Channels 2":i32[], "Name":string, "Reset Z":bool, "Record final Z":bool, "Auto Retract Status":bool, "Threshold":sgl, "Auto Retract Signal Index":i32, "Auto Retract Condition":bool}[]
  T2 = cluster{"Amplitude (mod. signal unit)":sgl, "Lockin on/off status":bool, "Advanced options":cluster{"Z-Controller Hold":bool, "Record final Z":bool, "Reset Bias":bool}, "Backward sweep":bool, "Number of points":i32, "Channels":string[], "Parameters":string[], "Fixed parameters":string[], "Multiple sweeps configuration":cluster{"Number of Sweeps":i32, "Save all":bool}, "Initialization":cluster{"Z averaging time (s)":sgl, "Z offset (m)":sgl, "Initial settling time (s)":sgl}, "Sweep Timing":cluster{"Max. slew rate (V/s)":sgl, "Settling time (s)":sgl, "Integration time (s)":sgl}, "End of Sweep":cluster{"End settling time (s)":sgl, "Z control time (s)":sgl}, "Start value (V)":sgl, "End value (V)":sgl, "Channels 2":i32[], "Name":string}[]
  T3 = enum32{"Page 1", "Page 2", "Page 3", "Page 4", "Page 5"}
  T4 = cluster{"Drift Correction Settings":cluster{"Drift Correction every":i32, "Drift correction Pixels":i32, "Channel index (0-23)":u8, "MaxImagesBack":i32, "Threshold":i32, "Increment":i32, "max applied Drift Correction":i32, "Correct Drift":bool, "Correlate":u16, "Correct z drift":bool, "zdrift \nDuration (s)":dbl}, "Spectroscopy Setting":cluster{"Imaging Current":dbl, "ref Current":dbl, "tip Speed (m/s)":sgl, "Imaging Bias":dbl, "ref Bias":dbl, "preSTS delay [ms]":u32, "STS z offset":dbl, "during Spec Bias (V)":sgl, "trigger1 < Hz":sgl, "trigger 2 >Hz":sgl, "autoStop":bool, "Spectroscopy":u16, "PLL ON/OFF":bool, "readjust setpoint every ":i32, "z Reference":bool, "Lock In":bool}, "Misc":cluster{"File name":string, "Email when finished":string}, "Grid Settings":cluster{"type":u16, "type order":u16, "X pixel":i32, "Y pixel":i32, "Grid_Parms":cluster{"center X (m)":sgl, "center Y (m)":sgl, "width (m)":sgl, "height (m)":sgl, "angle (deg)":sgl}}, "STS Param List #1 ":u16, "ZSpec Param List #1  ":u16, "Repeat Experiment":cluster{"Repeat":bool, "Repeat Parameter":u16, "Values List #1":i32}}
  T5 = cluster{"Drift Correction Settings":cluster{"Drift Correction every":i32, "Drift correction Pixels":i32, "Channel index (0-23)":u8, "MaxImagesBack":i32, "Threshold":i32, "Increment":i32, "max applied Drift Correction":i32, "Correct Drift":bool, "Correlate":u16, "Correct z drift":bool, "zdrift \nDuration (s)":dbl}, "Spectroscopy Setting":cluster{"Imaging Current":dbl, "ref Current":dbl, "tip Speed (m/s)":sgl, "Imaging Bias":dbl, "ref Bias":dbl, "preSTS delay [ms]":u32, "STS z offset":dbl, "during Spec Bias (V)":sgl, "trigger1 < Hz":sgl, "trigger 2 >Hz":sgl, "autoStop":bool, "Spectroscopy":u16, "PLL ON/OFF":bool, "readjust setpoint every ":i32, "z Reference":bool, "Lock In":bool}, "Misc":cluster{"File name":string, "Email when finished":string}, "Grid Settings":cluster{"type":u16, "type order":u16, "X pixel":i32, "Y pixel":i32, "Grid_Parms":cluster{"center X (m)":sgl, "center Y (m)":sgl, "width (m)":sgl, "height (m)":sgl, "angle (deg)":sgl}}, "STS Param List #2 ":u16, "ZSpec Param List  #2 ":u16, "Repeat Experiment":cluster{"Repeat":bool, "Repeat Parameter":u16, "Values List #2":i32}}
  T6 = cluster{"Drift Correction Settings":cluster{"Drift Correction every":i32, "Drift correction Pixels":i32, "Channel index (0-23)":u8, "MaxImagesBack":i32, "Threshold":i32, "Increment":i32, "max applied Drift Correction":i32, "Correct Drift":bool, "Correlate":u16, "Correct z drift":bool, "zdrift \nDuration (s)":dbl}, "Spectroscopy Setting":cluster{"Imaging Current":dbl, "ref Current":dbl, "tip Speed (m/s)":sgl, "Imaging Bias":dbl, "ref Bias":dbl, "preSTS delay [ms]":u32, "STS z offset":dbl, "during Spec Bias (V)":sgl, "trigger1 < Hz":sgl, "trigger 2 >Hz":sgl, "autoStop":bool, "Spectroscopy":u16, "PLL ON/OFF":bool, "readjust setpoint every ":i32, "z Reference":bool, "Lock In":bool}, "Misc":cluster{"File name":string, "Email when finished":string}, "Grid Settings":cluster{"type":u16, "type order":u16, "X pixel":i32, "Y pixel":i32, "Grid_Parms":cluster{"center X (m)":sgl, "center Y (m)":sgl, "width (m)":sgl, "height (m)":sgl, "angle (deg)":sgl}}, "STS Param List #3 ":u16, "ZSpec Param List #3 ":u16, "Repeat Experiment":cluster{"Repeat":bool, "Repeat Parameter":u16, "Values List #3":i32}}
  T7 = cluster{"Drift Correction Settings":cluster{"Drift Correction every":i32, "Drift correction Pixels":i32, "Channel index (0-23)":u8, "MaxImagesBack":i32, "Threshold":i32, "Increment":i32, "max applied Drift Correction":i32, "Correct Drift":bool, "Correlate":u16, "Correct z drift":bool, "zdrift \nDuration (s)":dbl}, "Spectroscopy Setting":cluster{"Imaging Current":dbl, "ref Current":dbl, "tip Speed (m/s)":sgl, "Imaging Bias":dbl, "ref Bias":dbl, "preSTS delay [ms]":u32, "STS z offset":dbl, "during Spec Bias (V)":sgl, "trigger1 < Hz":sgl, "trigger 2 >Hz":sgl, "autoStop":bool, "Spectroscopy":u16, "PLL ON/OFF":bool, "readjust setpoint every ":i32, "z Reference":bool, "Lock In":bool}, "Misc":cluster{"File name":string, "Email when finished":string}, "Grid Settings":cluster{"type":u16, "type order":u16, "X pixel":i32, "Y pixel":i32, "Grid_Parms":cluster{"center X (m)":sgl, "center Y (m)":sgl, "width (m)":sgl, "height (m)":sgl, "angle (deg)":sgl}}, "STS Param List #4 ":u16, "ZSpec Param List  #4":u16, "Repeat Experiment":cluster{"Repeat":bool, "Repeat Parameter":u16, "Values List #4":i32}}
  T8 = cluster{"Drift Correction Settings":cluster{"Drift Correction every":i32, "Drift correction Pixels":i32, "Channel index (0-23)":u8, "MaxImagesBack":i32, "Threshold":i32, "Increment":i32, "max applied Drift Correction":i32, "Correct Drift":bool, "Correlate":u16, "Correct z drift":bool, "zdrift \nDuration (s)":dbl}, "Spectroscopy Setting":cluster{"Imaging Current":dbl, "ref Current":dbl, "tip Speed (m/s)":sgl, "Imaging Bias":dbl, "ref Bias":dbl, "preSTS delay [ms]":u32, "STS z offset":dbl, "during Spec Bias (V)":sgl, "trigger1 < Hz":sgl, "trigger 2 >Hz":sgl, "autoStop":bool, "Spectroscopy":u16, "PLL ON/OFF":bool, "readjust setpoint every ":i32, "z Reference":bool, "Lock In":bool}, "Misc":cluster{"File name":string, "Email when finished":string}, "Grid Settings":cluster{"type":u16, "type order":u16, "X pixel":i32, "Y pixel":i32, "Grid_Parms":cluster{"center X (m)":sgl, "center Y (m)":sgl, "width (m)":sgl, "height (m)":sgl, "angle (deg)":sgl}}, "STS Param List #5 ":u16, "ZSpec Param List #5  ":u16, "Repeat Experiment":cluster{"Repeat":bool, "Repeat Parameter":u16, "Values List #5":i32}}
  T9 = cluster{"Amplitude (mod. signal unit)":sgl, "Lockin on/off status":bool, "Backward sweep":bool, "Number of points":i32, "Channels":string[], "Parameters":string[], "Fixed parameters":string[], "Multiple sweeps configuration":cluster{"Number of Sweeps":i32, "Save all":bool}, "Initialization":cluster{"Z averaging time (s)":sgl, "Initial settling time (s)":sgl}, "Sweep Timing":cluster{"Max. slew rate (V/s)":sgl, "Settling time (s)":sgl, "Integration time (s)":sgl}, "End of Sweep":cluster{"End settling time (s)":sgl, "Z control time (s)":sgl}, "Initial Z-Offset (m)":sgl, "Sweep Distance (m)":sgl, "Channels 2":i32[], "Name":string, "Reset Z":bool, "Record final Z":bool, "Auto Retract Status":bool, "Threshold":sgl, "Auto Retract Signal Index":i32, "Auto Retract Condition":bool}
  T10 = cluster{"Amplitude (mod. signal unit)":sgl, "Lockin on/off status":bool, "Advanced options":cluster{"Z-Controller Hold":bool, "Record final Z":bool, "Reset Bias":bool}, "Backward sweep":bool, "Number of points":i32, "Channels":string[], "Parameters":string[], "Fixed parameters":string[], "Multiple sweeps configuration":cluster{"Number of Sweeps":i32, "Save all":bool}, "Initialization":cluster{"Z averaging time (s)":sgl, "Z offset (m)":sgl, "Initial settling time (s)":sgl}, "Sweep Timing":cluster{"Max. slew rate (V/s)":sgl, "Settling time (s)":sgl, "Integration time (s)":sgl}, "End of Sweep":cluster{"End settling time (s)":sgl, "Z control time (s)":sgl}, "Start value (V)":sgl, "End value (V)":sgl, "Channels 2":i32[], "Name":string}
  T11 = cluster{"Drift Correction every":i32, "Drift correction Pixels":i32, "Channel index (0-23)":u8, "MaxImagesBack":i32, "Threshold":i32, "Increment":i32, "max applied Drift Correction":i32, "Correct Drift":bool, "Correlate":u16, "Correct z drift":bool, "zdrift \nDuration (s)":dbl}
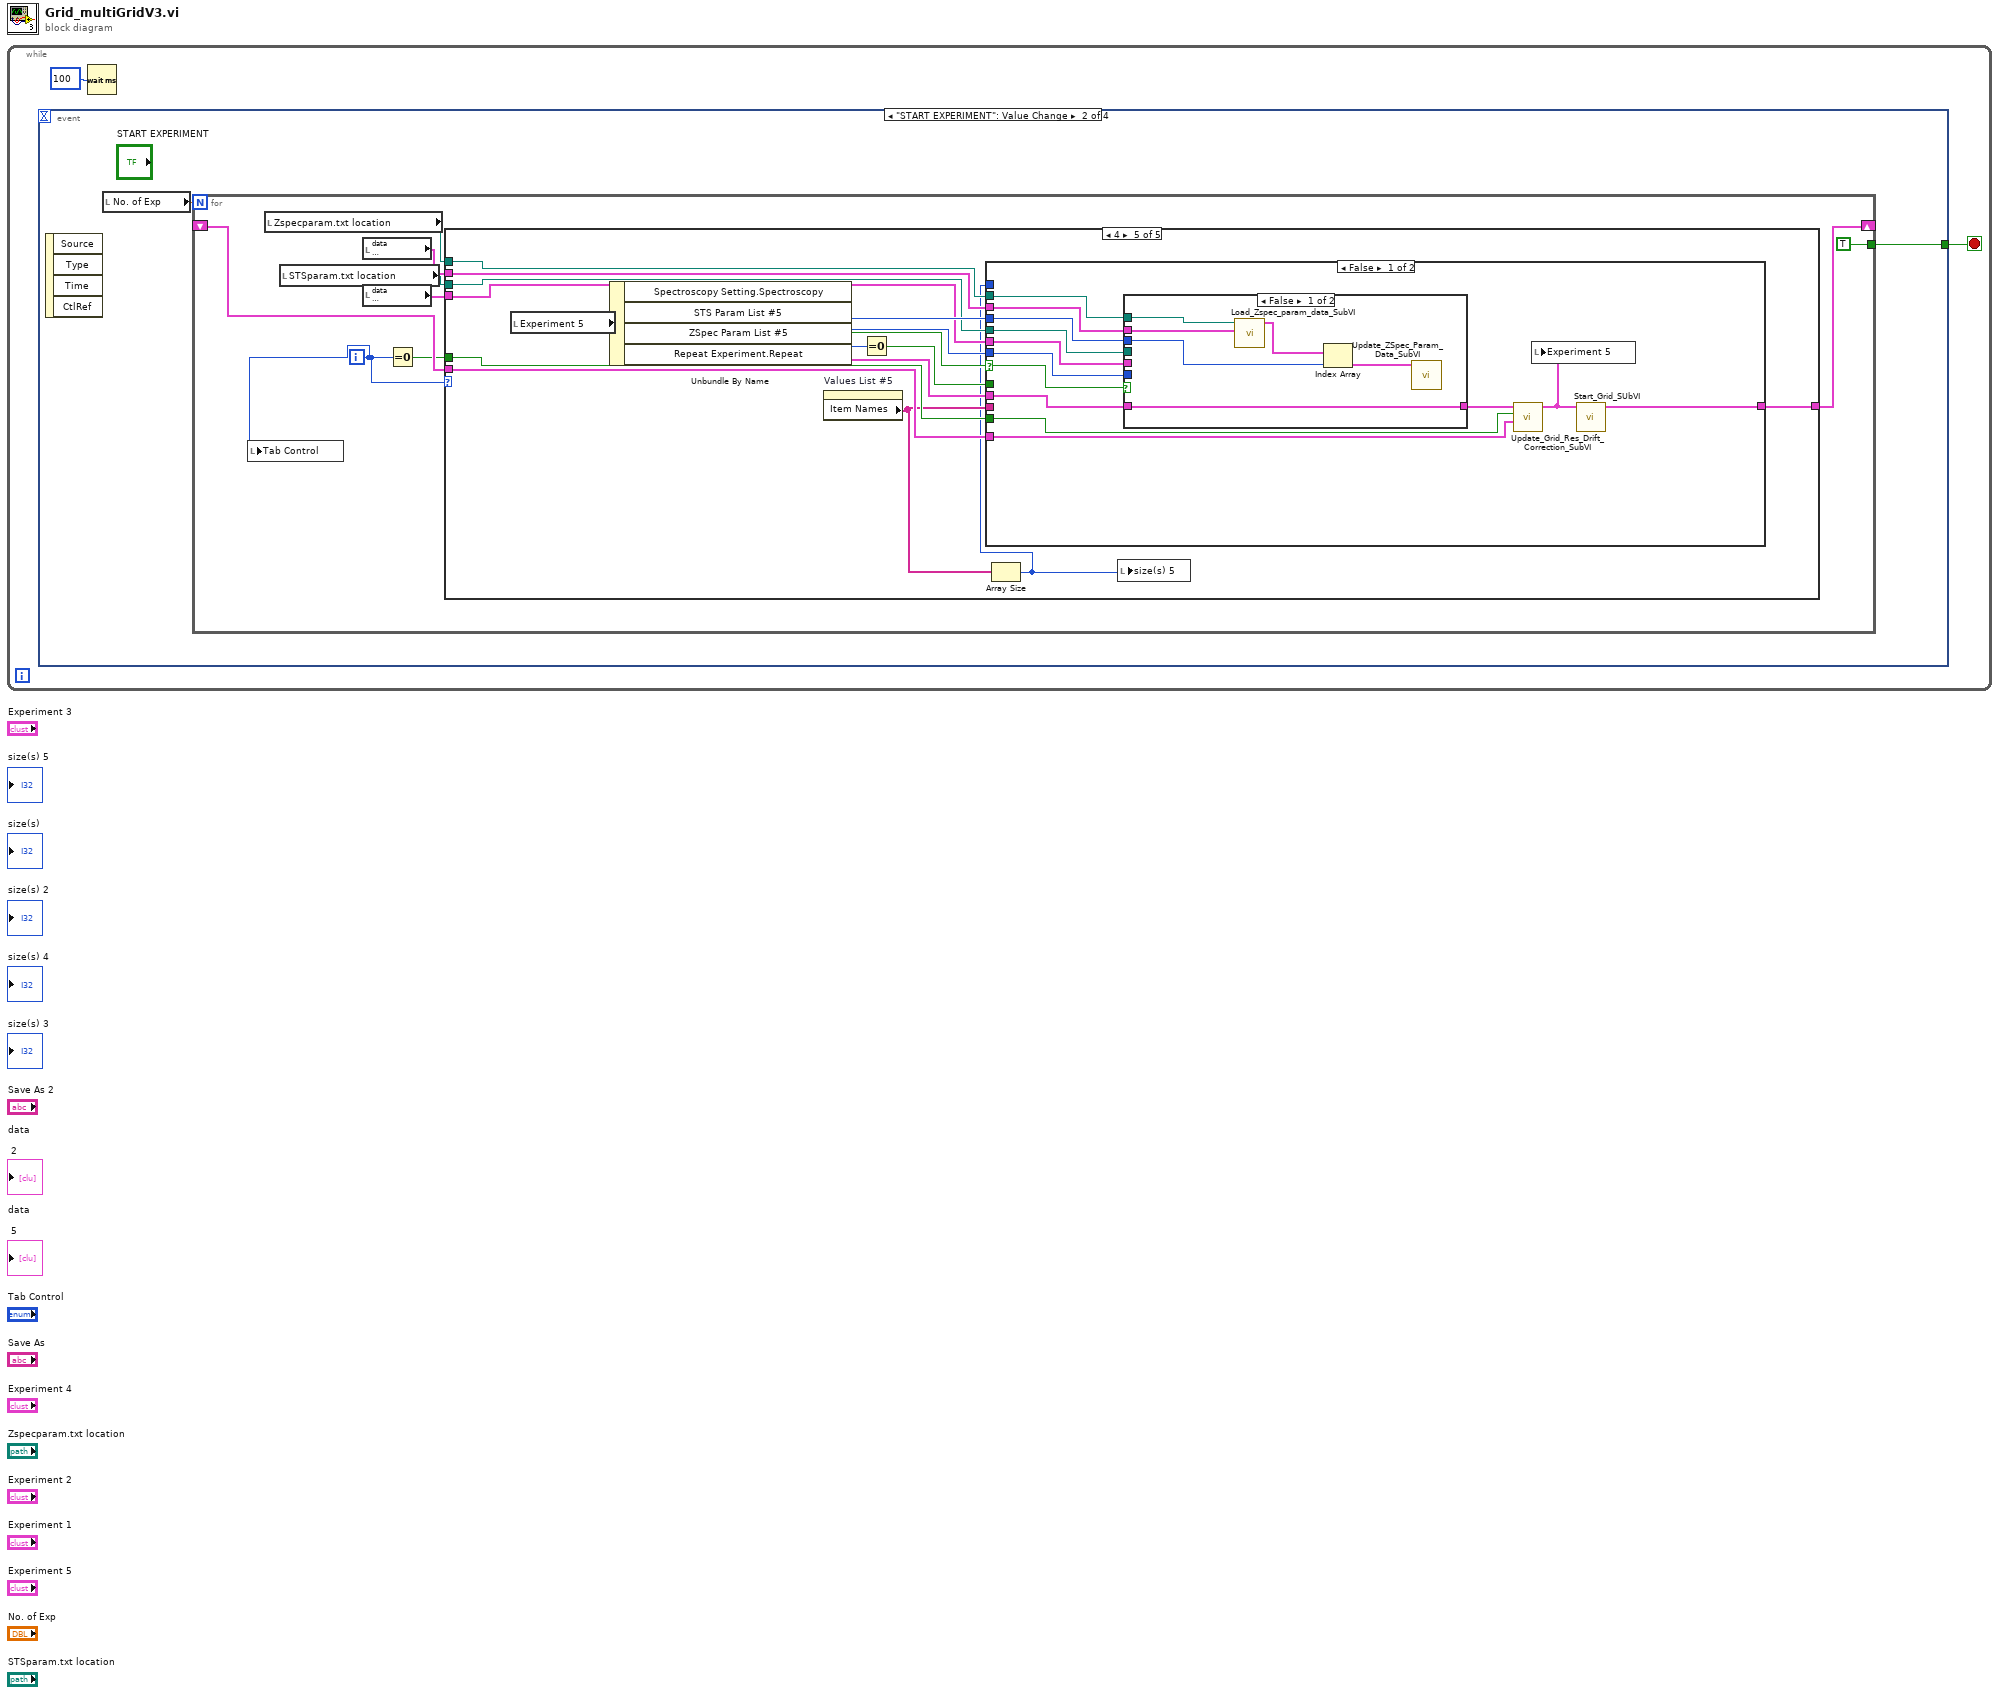
[diagram p0: block diagram]
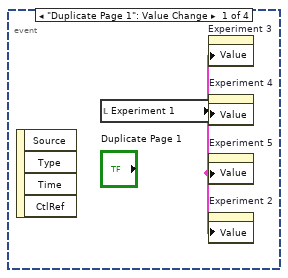
[diagram p2: hidden frame]
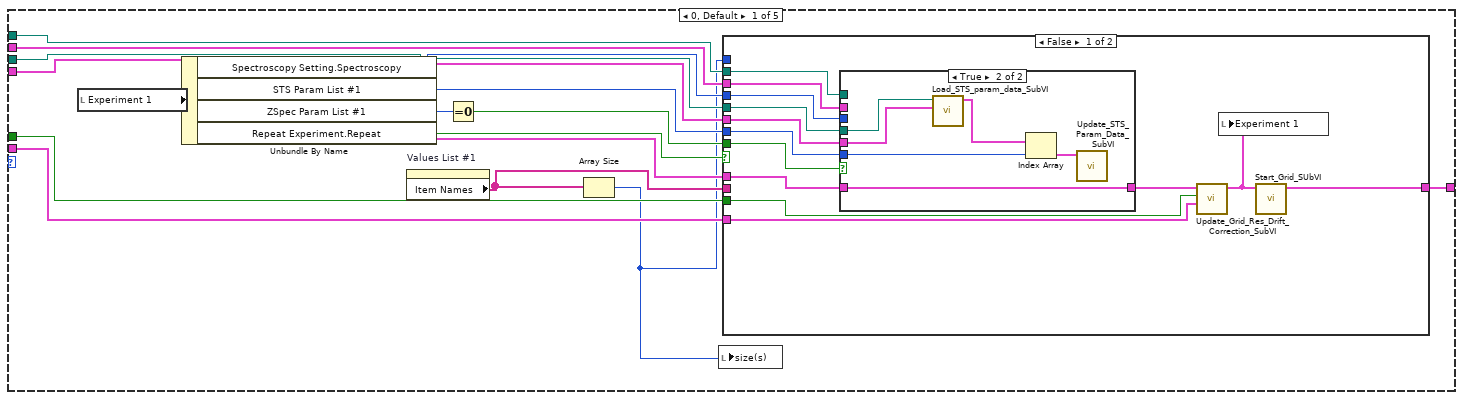
[diagram p3: hidden frame]
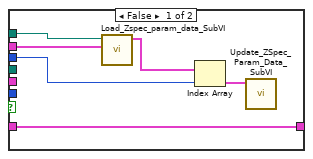
[diagram p4: hidden frame]
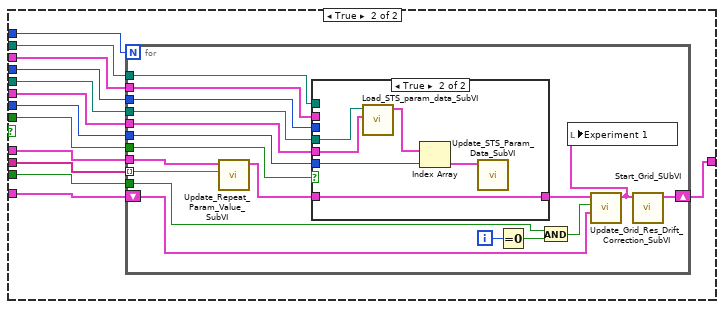
[diagram p5: hidden frame]
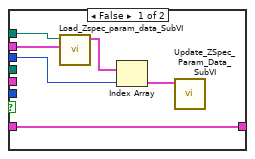
[diagram p6: hidden frame]
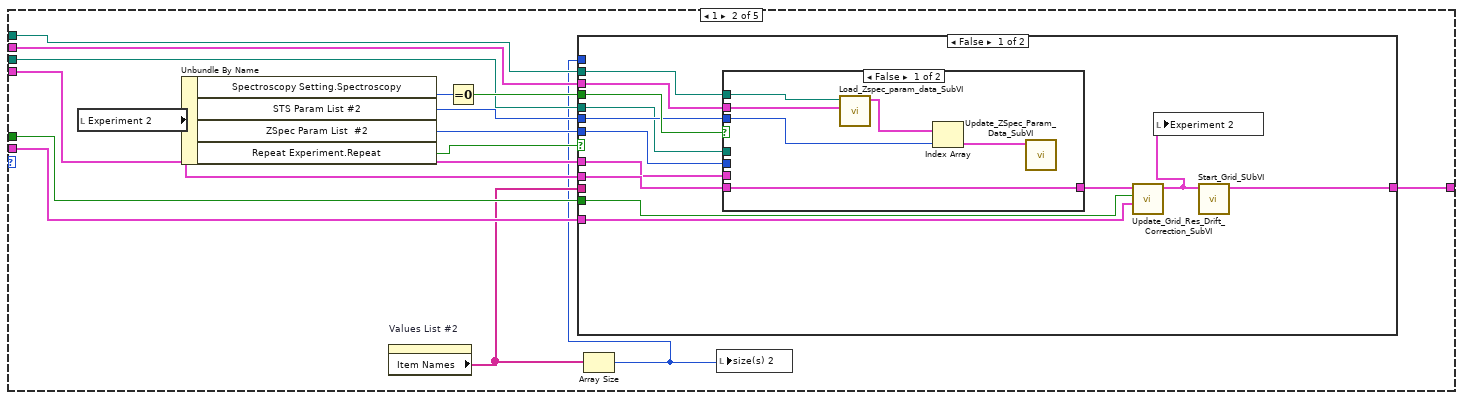
[diagram p7: hidden frame]
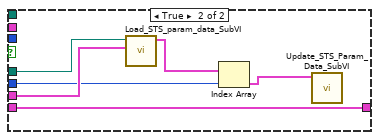
[diagram p8: hidden frame]
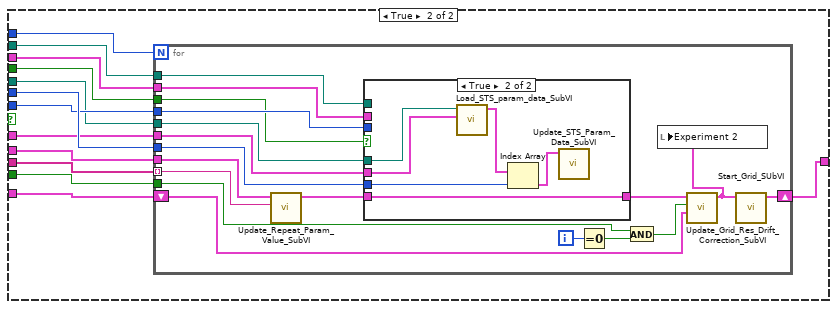
[diagram p9: hidden frame]
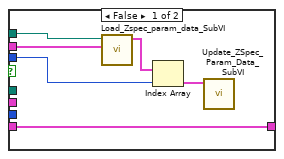
[diagram p10: hidden frame]
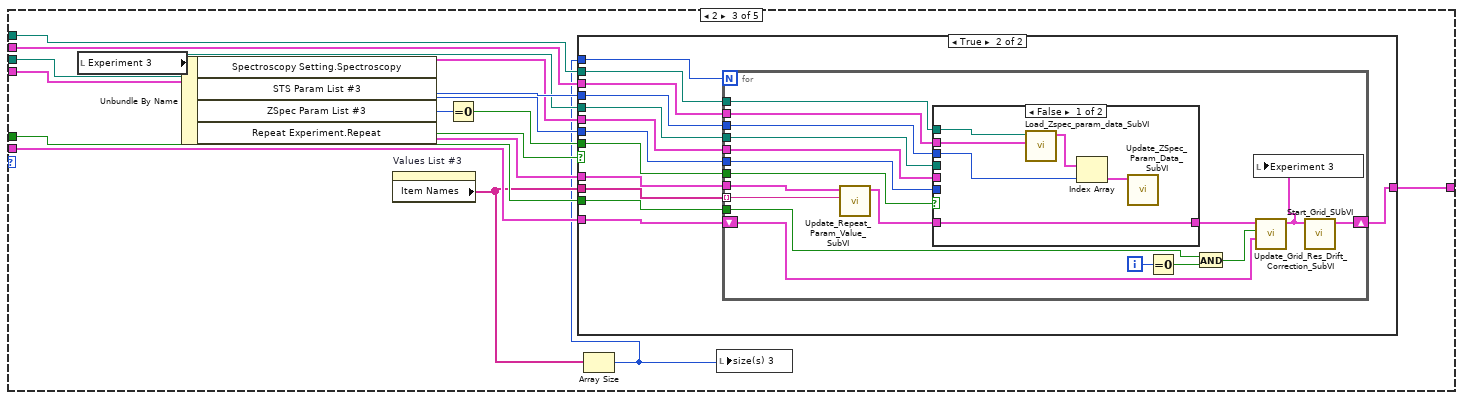
[diagram p11: hidden frame]
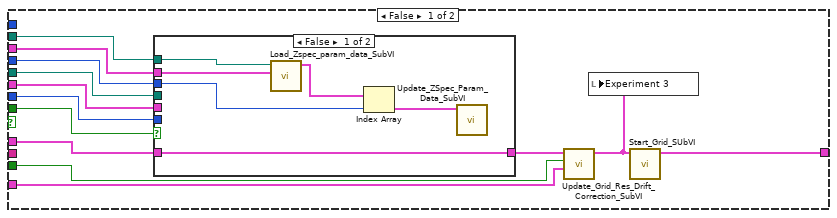
[diagram p12: hidden frame]
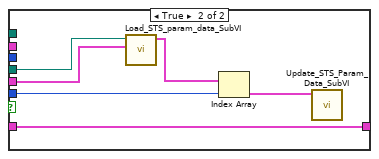
[diagram p13: hidden frame]
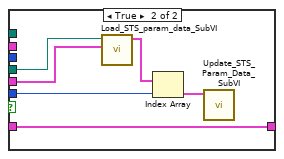
[diagram p14: hidden frame]
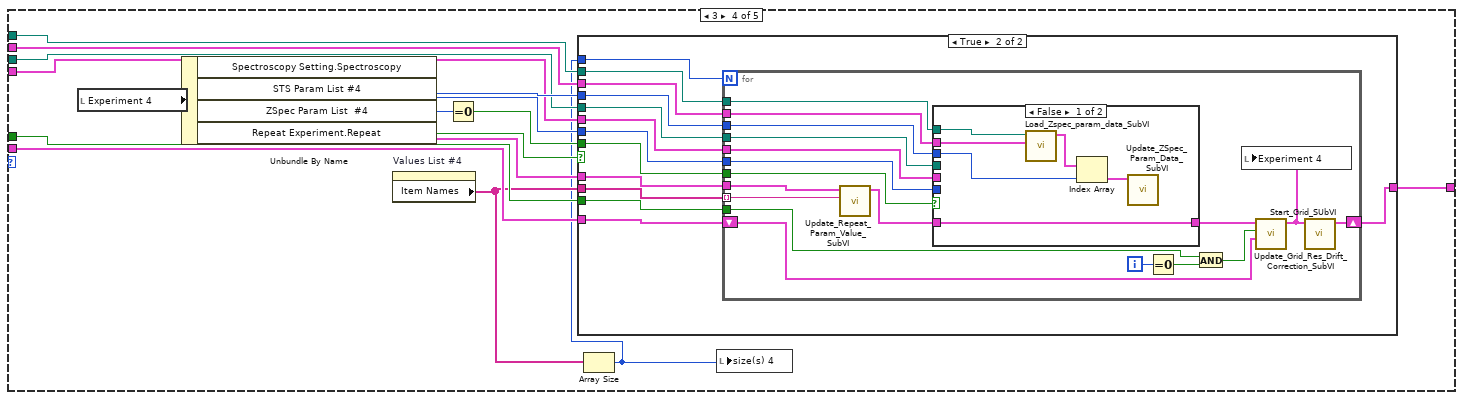
[diagram p15: hidden frame]
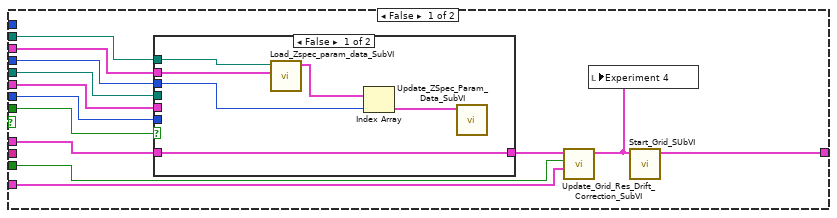
[diagram p16: hidden frame]
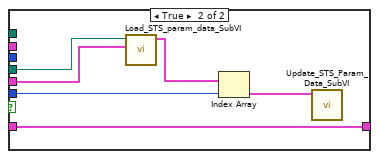
[diagram p17: hidden frame]
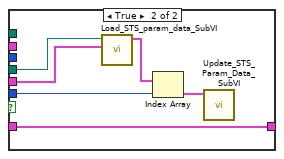
[diagram p18: hidden frame]
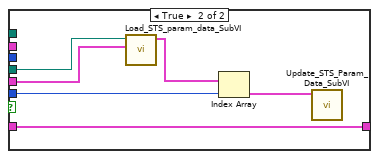
[diagram p19: hidden frame]
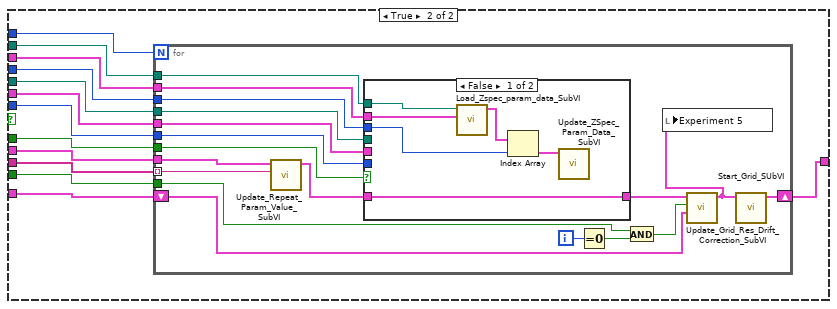
[diagram p20: hidden frame]
diagram:
  n1 = while {
    stop <- w2 stop-if-true
    n2 = event shown="[1] \"START EXPERIMENT\": Value Change" {
      selector: _ -> [_ _ _ _]
      dyn-events: _ -> [_ _ _ _]
      timeout: _ -> [_ _ _ _]
      tunnel: [_ w5 _ "stop"] -> w2
      event "Duplicate Page 1": Value Change {
        n3 = event-data() -> ()  [unwired: 1 in, 4 out]
        n4 = local read "Experiment 1"() -> (w3:T4)
        n5 = property on="Experiment 3" class="Clust (strict)"("Value"=w3) -> ()  [unwired: 2 in, 2 out]
        n6 = property on="Experiment 4" class="Clust (strict)"("Value"=w3) -> ()  [unwired: 2 in, 2 out]
        n7 = property on="Experiment 5" class="Clust (strict)"("Value"=w3) -> ()  [unwired: 2 in, 2 out]
        n8 = property on="Experiment 2" class="Clust (strict)"("Value"=w3) -> ()  [unwired: 2 in, 2 out]
      }
      event "START EXPERIMENT": Value Change {
        n9 = event-data() -> ()  [unwired: 1 in, 4 out]
        n10 = local read "No. of Exp"() -> (w4:dbl)
        n11 = for {
          N: w4 -> [_]
          shift-right: [w11] -> _
          shift-left: _ -> [w13]
          tunnel: [TRUE] -> w5
          i -> [w6]
          n12 = local write "Tab Control"(w6) -> ()
          n13 = local read "Zspecparam.txt location"() -> (w10:path)
          n14 = local read "STSparam.txt location"() -> (w9:path)
          n15 = local read "data\n\n 5"() -> (w7:T1)
          n16 = local read "data\n\n 2"() -> (w8:T2)
          n17 = Equal To 0?(x=w6) -> (x = 0?=w12:bool)
          n18 = case shown="4" w6 {
            tunnel: [w29 w112 w188 w278 w361] -> w11
            tunnel: w13 -> [w23 w106 w191 w275 w360]
            tunnel: w12 -> [w22 w105 w192 w276 w359]
            tunnel: w10 -> [w18 w99 w182 w268 w350]
            tunnel: w9 -> [w19 w100 w183 w267 w351]
            tunnel: w8 -> [w17 w101 w184 w266 w349]
            tunnel: w7 -> [w16 w102 w185 w265 w348]
            frame 0, Default {
              n19 = local read "Experiment 1"() -> (w26:T4)
              n20 = Unbundle By Name(w26) -> ("Spectroscopy Setting.Spectroscopy"=w27:u16, "STS Param List #1"=w25:u16, "ZSpec Param List #1"=w24:u16, "Repeat Experiment.Repeat"=w20:bool)
              n21 = property on="Values List #1" class="LstBox (strict)"() -> ("Item Names"=w21:string[])  [unwired: 2 in, 2 out]
              n22 = Equal To 0?(x=w27) -> (x = 0?=w28:bool)
              n23 = Array Size(array=w21) -> (size(s)=w15:i32)
              n24 = local write "size(s)"(w15) -> ()
              n25 = case shown="False" w20 {
                tunnel: w15 -> [_ w67]
                tunnel: w26 -> [w38 w66]
                tunnel: w28 -> [w35 w65]
                tunnel: w25 -> [w39 w64]
                tunnel: w24 -> [w36 w63]
                tunnel: [w42 w62] -> w29
                tunnel: w23 -> [w41 w61]
                tunnel: w22 -> [w40 w60]
                tunnel: w21 -> [_ w59]
                tunnel: w19 -> [w32 w58]
                tunnel: w18 -> [w33 w57]
                tunnel: w17 -> [w31 w56]
                tunnel: w16 -> [w34 w55]
                frame False {
                  n26 = case shown="True" w35 {
                    tunnel: w39 -> [_ w53]
                    tunnel: w31 -> [_ w52]
                    tunnel: w32 -> [_ w51]
                    tunnel: w38 -> [w45 w49]
                    tunnel: [w45 w49] -> w37
                    tunnel: w34 -> [w47 _]
                    tunnel: w33 -> [w46 _]
                    tunnel: w36 -> [w43 _]
                    frame False {
                      n27 = call "Load_Zspec_param_data_SubVI.vi"("data\n\n 5"=w47, "Zspecparam.txt location"=w46) -> ("data"=w44:T1)  [unwired: 9 in]
                      n28 = Index Array(array=w44, index=w43) -> (element=w48:T9)
                      n29 = call "Update_ZSpec_Param_Data_SubVI.vi"("output cluster"=w48) -> ()  [unwired: 11 in]
                    }
                    frame True {
                      n30 = call "Load_STS_param_data_SubVI.vi"("data\n\n in"=w52, "STSparam.txt location"=w51) -> ("data\n\n out"=w50:T2)  [unwired: 9 in]
                      n31 = Index Array(array=w50, index=w53) -> (element=w54:T10)
                      n32 = call "Update_STS_Param_Data_SubVI.vi"("STSparameters"=w54) -> ()  [unwired: 11 in]
                    }
                  }
                  n33 = call "Update_Grid_Res_Drift_Correction_SubVI.vi"("Drift Correction Settings"=w41, "Boolean"=w40, "Experiment 6"=w37) -> ("Experiment 5"=w30:T8)  [unwired: 8 in]
                  n34 = local write "Experiment 1"(w30) -> ()
                  n35 = call "Start_Grid_SUbVI.vi"("Experiment 5"=w30) -> ("Drift Correction Settings"=w42:T11)  [unwired: 10 in]
                }
                frame True {
                  n36 = for {
                    N: w67 -> [_]
                    tunnel: w59 -> [w85] mode=indexing
                    tunnel: w66 -> [w84]
                    tunnel: w65 -> [w73]
                    tunnel: w64 -> [w75]
                    tunnel: w63 -> [w74]
                    shift-right: [w79] -> w62
                    shift-left: w61 -> [w83]
                    tunnel: w60 -> [w78]
                    tunnel: w58 -> [w72]
                    tunnel: w57 -> [w71]
                    tunnel: w56 -> [w70]
                    tunnel: w55 -> [w69]
                    i -> [w82]
                    n37 = call "Update_Repeat_Param_Value_SubVI.vi"("String"=w85, "Experiment 6"=w84) -> ("Experiment 5"=w76:T8)  [unwired: 9 in]
                    n38 = case shown="True" w73 {
                      tunnel: w75 -> [_ w96]
                      tunnel: w70 -> [_ w95]
                      tunnel: w72 -> [_ w94]
                      tunnel: w76 -> [w88 w93]
                      tunnel: [w88 w93] -> w77
                      tunnel: w69 -> [w90 _]
                      tunnel: w71 -> [w89 _]
                      tunnel: w74 -> [w86 _]
                      frame False {
                        n39 = call "Load_Zspec_param_data_SubVI.vi"("data\n\n 5"=w90, "Zspecparam.txt location"=w89) -> ("data"=w87:T1)  [unwired: 9 in]
                        n40 = Index Array(array=w87, index=w86) -> (element=w91:T9)
                        n41 = call "Update_ZSpec_Param_Data_SubVI.vi"("output cluster"=w91) -> ()  [unwired: 11 in]
                      }
                      frame True {
                        n42 = call "Load_STS_param_data_SubVI.vi"("data\n\n in"=w95, "STSparam.txt location"=w94) -> ("data\n\n out"=w92:T2)  [unwired: 9 in]
                        n43 = Index Array(array=w92, index=w96) -> (element=w97:T10)
                        n44 = call "Update_STS_Param_Data_SubVI.vi"("STSparameters"=w97) -> ()  [unwired: 11 in]
                      }
                    }
                    n45 = Equal To 0?(x=w82) -> (x = 0?=w81:bool)
                    n46 = And(x=w78, y=w81) -> (x .and. y?=w80:bool)
                    n47 = call "Update_Grid_Res_Drift_Correction_SubVI.vi"("Drift Correction Settings"=w83, "Boolean"=w80, "Experiment 6"=w77) -> ("Experiment 5"=w68:T8)  [unwired: 8 in]
                    n48 = local write "Experiment 1"(w68) -> ()
                    n49 = call "Start_Grid_SUbVI.vi"("Experiment 5"=w68) -> ("Drift Correction Settings"=w79:T11)  [unwired: 10 in]
                  }
                }
              }
            }
            frame 1 {
              n50 = local read "Experiment 2"() -> (w104:T5)
              n51 = Unbundle By Name(w104) -> ("Spectroscopy Setting.Spectroscopy"=w111:u16, "STS Param List #2"=w109:u16, "ZSpec Param List  #2"=w108:u16, "Repeat Experiment.Repeat"=w107:bool)
              n52 = property on="Values List #2" class="LstBox (strict)"() -> ("Item Names"=w103:string[])  [unwired: 2 in, 2 out]
              n53 = Equal To 0?(x=w111) -> (x = 0?=w110:bool)
              n54 = Array Size(array=w103) -> (size(s)=w98:i32)
              n55 = case shown="False" w107 {
                tunnel: w98 -> [_ w150]
                tunnel: w104 -> [w120 w149]
                tunnel: w110 -> [w122 w148]
                tunnel: w109 -> [w121 w147]
                tunnel: w108 -> [w118 w146]
                tunnel: [w125 w145] -> w112
                tunnel: w106 -> [w124 w144]
                tunnel: w105 -> [w123 w143]
                tunnel: w103 -> [_ w142]
                tunnel: w102 -> [w114 w141]
                tunnel: w101 -> [w115 w140]
                tunnel: w100 -> [w117 w139]
                tunnel: w99 -> [w116 w138]
                frame False {
                  n56 = case shown="False" w122 {
                    tunnel: w121 -> [w130 _]
                    tunnel: w115 -> [_ w136]
                    tunnel: w117 -> [_ w135]
                    tunnel: w120 -> [w127 w133]
                    tunnel: [w127 w133] -> w119
                    tunnel: w114 -> [w129 _]
                    tunnel: w116 -> [w128 _]
                    tunnel: w118 -> [_ w132]
                    frame False {
                      n57 = call "Load_Zspec_param_data_SubVI.vi"("data\n\n 5"=w129, "Zspecparam.txt location"=w128) -> ("data"=w126:T1)  [unwired: 9 in]
                      n58 = Index Array(array=w126, index=w130) -> (element=w131:T9)
                      n59 = call "Update_ZSpec_Param_Data_SubVI.vi"("output cluster"=w131) -> ()  [unwired: 11 in]
                    }
                    frame True {
                      n60 = call "Load_STS_param_data_SubVI.vi"("data\n\n in"=w136, "STSparam.txt location"=w135) -> ("data\n\n out"=w134:T2)  [unwired: 9 in]
                      n61 = Index Array(array=w134, index=w132) -> (element=w137:T10)
                      n62 = call "Update_STS_Param_Data_SubVI.vi"("STSparameters"=w137) -> ()  [unwired: 11 in]
                    }
                  }
                  n63 = call "Update_Grid_Res_Drift_Correction_SubVI.vi"("Drift Correction Settings"=w124, "Boolean"=w123, "Experiment 6"=w119) -> ("Experiment 5"=w113:T8)  [unwired: 8 in]
                  n64 = local write "Experiment 2"(w113) -> ()
                  n65 = call "Start_Grid_SUbVI.vi"("Experiment 5"=w113) -> ("Drift Correction Settings"=w125:T11)  [unwired: 10 in]
                }
                frame True {
                  n66 = for {
                    N: w150 -> [_]
                    tunnel: w142 -> [w168] mode=indexing
                    tunnel: w149 -> [w167]
                    tunnel: w148 -> [w158]
                    tunnel: w147 -> [w160]
                    tunnel: w146 -> [w159]
                    shift-right: [w162] -> w145
                    shift-left: w144 -> [w166]
                    tunnel: w143 -> [w161]
                    tunnel: w141 -> [w155]
                    tunnel: w140 -> [w154]
                    tunnel: w139 -> [w153]
                    tunnel: w138 -> [w152]
                    i -> [w165]
                    n67 = call "Update_Repeat_Param_Value_SubVI.vi"("String"=w168, "Experiment 6"=w167) -> ("Experiment 5"=w157:T8)  [unwired: 9 in]
                    n68 = case shown="True" w158 {
                      tunnel: w160 -> [_ w179]
                      tunnel: w154 -> [_ w178]
                      tunnel: w153 -> [_ w177]
                      tunnel: w157 -> [w171 w176]
                      tunnel: [w171 w176] -> w156
                      tunnel: w155 -> [w173 _]
                      tunnel: w152 -> [w172 _]
                      tunnel: w159 -> [w169 _]
                      frame False {
                        n69 = call "Load_Zspec_param_data_SubVI.vi"("data\n\n 5"=w173, "Zspecparam.txt location"=w172) -> ("data"=w170:T1)  [unwired: 9 in]
                        n70 = Index Array(array=w170, index=w169) -> (element=w174:T9)
                        n71 = call "Update_ZSpec_Param_Data_SubVI.vi"("output cluster"=w174) -> ()  [unwired: 11 in]
                      }
                      frame True {
                        n72 = call "Load_STS_param_data_SubVI.vi"("data\n\n in"=w178, "STSparam.txt location"=w177) -> ("data\n\n out"=w175:T2)  [unwired: 9 in]
                        n73 = Index Array(array=w175, index=w179) -> (element=w180:T10)
                        n74 = call "Update_STS_Param_Data_SubVI.vi"("STSparameters"=w180) -> ()  [unwired: 11 in]
                      }
                    }
                    n75 = Equal To 0?(x=w165) -> (x = 0?=w164:bool)
                    n76 = And(x=w161, y=w164) -> (x .and. y?=w163:bool)
                    n77 = call "Update_Grid_Res_Drift_Correction_SubVI.vi"("Drift Correction Settings"=w166, "Boolean"=w163, "Experiment 6"=w156) -> ("Experiment 5"=w151:T8)  [unwired: 8 in]
                    n78 = local write "Experiment 2"(w151) -> ()
                    n79 = call "Start_Grid_SUbVI.vi"("Experiment 5"=w151) -> ("Drift Correction Settings"=w162:T11)  [unwired: 10 in]
                  }
                }
              }
              n80 = local write "size(s) 2"(w98) -> ()
            }
            frame 2 {
              n81 = local read "Experiment 3"() -> (w189:T6)
              n82 = Unbundle By Name(w189) -> ("Spectroscopy Setting.Spectroscopy"=w186:u16, "STS Param List #3"=w195:u16, "ZSpec Param List #3"=w194:u16, "Repeat Experiment.Repeat"=w193:bool)
              n83 = property on="Values List #3" class="LstBox (strict)"() -> ("Item Names"=w190:string[])  [unwired: 2 in, 2 out]
              n84 = Equal To 0?(x=w186) -> (x = 0?=w187:bool)
              n85 = Array Size(array=w190) -> (size(s)=w181:i32)
              n86 = case shown="True" w193 {
                tunnel: w181 -> [_ w233]
                tunnel: w189 -> [w204 w232]
                tunnel: w187 -> [w201 w231]
                tunnel: w195 -> [w203 w230]
                tunnel: w194 -> [w202 w229]
                tunnel: [w206 w228] -> w188
                tunnel: w191 -> [w208 w227]
                tunnel: w192 -> [w207 w226]
                tunnel: w190 -> [_ w225]
                tunnel: w185 -> [w200 w221]
                tunnel: w184 -> [w199 w224]
                tunnel: w183 -> [w198 w222]
                tunnel: w182 -> [w197 w223]
                frame False {
                  n87 = case shown="False" w201 {
                    tunnel: w203 -> [_ w219]
                    tunnel: w199 -> [_ w218]
                    tunnel: w198 -> [_ w217]
                    tunnel: w204 -> [w211 w216]
                    tunnel: [w211 w216] -> w205
                    tunnel: w200 -> [w213 _]
                    tunnel: w197 -> [w212 _]
                    tunnel: w202 -> [w209 _]
                    frame False {
                      n88 = call "Load_Zspec_param_data_SubVI.vi"("data\n\n 5"=w213, "Zspecparam.txt location"=w212) -> ("data"=w210:T1)  [unwired: 9 in]
                      n89 = Index Array(array=w210, index=w209) -> (element=w214:T9)
                      n90 = call "Update_ZSpec_Param_Data_SubVI.vi"("output cluster"=w214) -> ()  [unwired: 11 in]
                    }
                    frame True {
                      n91 = call "Load_STS_param_data_SubVI.vi"("data\n\n in"=w218, "STSparam.txt location"=w217) -> ("data\n\n out"=w215:T2)  [unwired: 9 in]
                      n92 = Index Array(array=w215, index=w219) -> (element=w220:T10)
                      n93 = call "Update_STS_Param_Data_SubVI.vi"("STSparameters"=w220) -> ()  [unwired: 11 in]
                    }
                  }
                  n94 = call "Update_Grid_Res_Drift_Correction_SubVI.vi"("Drift Correction Settings"=w208, "Boolean"=w207, "Experiment 6"=w205) -> ("Experiment 5"=w196:T8)  [unwired: 8 in]
                  n95 = local write "Experiment 3"(w196) -> ()
                  n96 = call "Start_Grid_SUbVI.vi"("Experiment 5"=w196) -> ("Drift Correction Settings"=w206:T11)  [unwired: 10 in]
                }
                frame True {
                  n97 = for {
                    N: w233 -> [_]
                    tunnel: w225 -> [w251] mode=indexing
                    tunnel: w232 -> [w250]
                    tunnel: w231 -> [w239]
                    tunnel: w230 -> [w241]
                    tunnel: w229 -> [w240]
                    shift-right: [w245] -> w228
                    shift-left: w227 -> [w249]
                    tunnel: w226 -> [w244]
                    tunnel: w224 -> [w238]
                    tunnel: w223 -> [w237]
                    tunnel: w222 -> [w236]
                    tunnel: w221 -> [w235]
                    i -> [w248]
                    n98 = call "Update_Repeat_Param_Value_SubVI.vi"("String"=w251, "Experiment 6"=w250) -> ("Experiment 5"=w243:T8)  [unwired: 9 in]
                    n99 = case shown="False" w239 {
                      tunnel: w241 -> [_ w262]
                      tunnel: w238 -> [_ w261]
                      tunnel: w236 -> [_ w260]
                      tunnel: w243 -> [w254 w259]
                      tunnel: [w254 w259] -> w242
                      tunnel: w235 -> [w256 _]
                      tunnel: w237 -> [w255 _]
                      tunnel: w240 -> [w252 _]
                      frame False {
                        n100 = call "Load_Zspec_param_data_SubVI.vi"("data\n\n 5"=w256, "Zspecparam.txt location"=w255) -> ("data"=w253:T1)  [unwired: 9 in]
                        n101 = Index Array(array=w253, index=w252) -> (element=w257:T9)
                        n102 = call "Update_ZSpec_Param_Data_SubVI.vi"("output cluster"=w257) -> ()  [unwired: 11 in]
                      }
                      frame True {
                        n103 = call "Load_STS_param_data_SubVI.vi"("data\n\n in"=w261, "STSparam.txt location"=w260) -> ("data\n\n out"=w258:T2)  [unwired: 9 in]
                        n104 = Index Array(array=w258, index=w262) -> (element=w263:T10)
                        n105 = call "Update_STS_Param_Data_SubVI.vi"("STSparameters"=w263) -> ()  [unwired: 11 in]
                      }
                    }
                    n106 = Equal To 0?(x=w248) -> (x = 0?=w247:bool)
                    n107 = And(x=w244, y=w247) -> (x .and. y?=w246:bool)
                    n108 = call "Update_Grid_Res_Drift_Correction_SubVI.vi"("Drift Correction Settings"=w249, "Boolean"=w246, "Experiment 6"=w242) -> ("Experiment 5"=w234:T8)  [unwired: 8 in]
                    n109 = local write "Experiment 3"(w234) -> ()
                    n110 = call "Start_Grid_SUbVI.vi"("Experiment 5"=w234) -> ("Drift Correction Settings"=w245:T11)  [unwired: 10 in]
                  }
                }
              }
              n111 = local write "size(s) 3"(w181) -> ()
            }
            frame 3 {
              n112 = local read "Experiment 4"() -> (w273:T7)
              n113 = Unbundle By Name(w273) -> ("Spectroscopy Setting.Spectroscopy"=w270:u16, "STS Param List #4"=w271:u16, "ZSpec Param List  #4"=w272:u16, "Repeat Experiment.Repeat"=w277:bool)
              n114 = property on="Values List #4" class="LstBox (strict)"() -> ("Item Names"=w274:string[])  [unwired: 2 in, 2 out]
              n115 = Equal To 0?(x=w270) -> (x = 0?=w269:bool)
              n116 = Array Size(array=w274) -> (size(s)=w264:i32)
              n117 = case shown="True" w277 {
                tunnel: w264 -> [_ w316]
                tunnel: w273 -> [w287 w315]
                tunnel: w269 -> [w286 w314]
                tunnel: w271 -> [w285 w313]
                tunnel: w272 -> [w284 w312]
                tunnel: [w291 w311] -> w278
                tunnel: w275 -> [w290 w310]
                tunnel: w276 -> [w289 w309]
                tunnel: w274 -> [_ w308]
                tunnel: w268 -> [w282 w307]
                tunnel: w267 -> [w283 w306]
                tunnel: w266 -> [w281 w305]
                tunnel: w265 -> [w280 w304]
                frame False {
                  n118 = case shown="False" w286 {
                    tunnel: w285 -> [_ w302]
                    tunnel: w281 -> [_ w301]
                    tunnel: w283 -> [_ w300]
                    tunnel: w287 -> [w294 w299]
                    tunnel: [w294 w299] -> w288
                    tunnel: w280 -> [w296 _]
                    tunnel: w282 -> [w295 _]
                    tunnel: w284 -> [w292 _]
                    frame False {
                      n119 = call "Load_Zspec_param_data_SubVI.vi"("data\n\n 5"=w296, "Zspecparam.txt location"=w295) -> ("data"=w293:T1)  [unwired: 9 in]
                      n120 = Index Array(array=w293, index=w292) -> (element=w297:T9)
                      n121 = call "Update_ZSpec_Param_Data_SubVI.vi"("output cluster"=w297) -> ()  [unwired: 11 in]
                    }
                    frame True {
                      n122 = call "Load_STS_param_data_SubVI.vi"("data\n\n in"=w301, "STSparam.txt location"=w300) -> ("data\n\n out"=w298:T2)  [unwired: 9 in]
                      n123 = Index Array(array=w298, index=w302) -> (element=w303:T10)
                      n124 = call "Update_STS_Param_Data_SubVI.vi"("STSparameters"=w303) -> ()  [unwired: 11 in]
                    }
                  }
                  n125 = call "Update_Grid_Res_Drift_Correction_SubVI.vi"("Drift Correction Settings"=w290, "Boolean"=w289, "Experiment 6"=w288) -> ("Experiment 5"=w279:T8)  [unwired: 8 in]
                  n126 = local write "Experiment 4"(w279) -> ()
                  n127 = call "Start_Grid_SUbVI.vi"("Experiment 5"=w279) -> ("Drift Correction Settings"=w291:T11)  [unwired: 10 in]
                }
                frame True {
                  n128 = for {
                    N: w316 -> [_]
                    tunnel: w308 -> [w334] mode=indexing
                    tunnel: w315 -> [w333]
                    tunnel: w314 -> [w324]
                    tunnel: w313 -> [w323]
                    tunnel: w312 -> [w322]
                    shift-right: [w328] -> w311
                    shift-left: w310 -> [w332]
                    tunnel: w309 -> [w327]
                    tunnel: w307 -> [w321]
                    tunnel: w306 -> [w320]
                    tunnel: w305 -> [w319]
                    tunnel: w304 -> [w318]
                    i -> [w331]
                    n129 = call "Update_Repeat_Param_Value_SubVI.vi"("String"=w334, "Experiment 6"=w333) -> ("Experiment 5"=w326:T8)  [unwired: 9 in]
                    n130 = case shown="False" w324 {
                      tunnel: w323 -> [_ w345]
                      tunnel: w319 -> [_ w344]
                      tunnel: w320 -> [_ w343]
                      tunnel: w326 -> [w335 w341]
                      tunnel: w318 -> [w339 _]
                      tunnel: w321 -> [w338 _]
                      tunnel: w322 -> [w336 _]
                      tunnel: [w335 w341] -> w325
                      frame False {
                        n131 = call "Load_Zspec_param_data_SubVI.vi"("data\n\n 5"=w339, "Zspecparam.txt location"=w338) -> ("data"=w337:T1)  [unwired: 9 in]
                        n132 = Index Array(array=w337, index=w336) -> (element=w340:T9)
                        n133 = call "Update_ZSpec_Param_Data_SubVI.vi"("output cluster"=w340) -> ()  [unwired: 11 in]
                      }
                      frame True {
                        n134 = call "Load_STS_param_data_SubVI.vi"("data\n\n in"=w344, "STSparam.txt location"=w343) -> ("data\n\n out"=w342:T2)  [unwired: 9 in]
                        n135 = Index Array(array=w342, index=w345) -> (element=w346:T10)
                        n136 = call "Update_STS_Param_Data_SubVI.vi"("STSparameters"=w346) -> ()  [unwired: 11 in]
                      }
                    }
                    n137 = Equal To 0?(x=w331) -> (x = 0?=w330:bool)
                    n138 = And(x=w327, y=w330) -> (x .and. y?=w329:bool)
                    n139 = call "Update_Grid_Res_Drift_Correction_SubVI.vi"("Drift Correction Settings"=w332, "Boolean"=w329, "Experiment 6"=w325) -> ("Experiment 5"=w317:T8)  [unwired: 8 in]
                    n140 = local write "Experiment 4"(w317) -> ()
                    n141 = call "Start_Grid_SUbVI.vi"("Experiment 5"=w317) -> ("Drift Correction Settings"=w328:T11)  [unwired: 10 in]
                  }
                }
              }
              n142 = local write "size(s) 4"(w264) -> ()
            }
            frame 4 {
              n143 = local read "Experiment 5"() -> (w356:T8)
              n144 = Unbundle By Name(w356) -> ("Spectroscopy Setting.Spectroscopy"=w352:u16, "STS Param List #5"=w354:u16, "ZSpec Param List #5"=w355:u16, "Repeat Experiment.Repeat"=w358:bool)
              n145 = property on="Values List #5" class="LstBox (strict)"() -> ("Item Names"=w357:string[])  [unwired: 2 in, 2 out]
              n146 = Equal To 0?(x=w352) -> (x = 0?=w353:bool)
              n147 = Array Size(array=w357) -> (size(s)=w347:i32)
              n148 = case shown="False" w358 {
                selector: w358 -> [w369 _]
                tunnel: w347 -> [_ w399]
                tunnel: w356 -> [w367 w398]
                tunnel: w353 -> [_ w397]
                tunnel: w354 -> [w370 w396]
                tunnel: w355 -> [w371 w395]
                tunnel: [w374 w394] -> w361
                tunnel: w360 -> [w373 w393]
                tunnel: w359 -> [w372 w392]
                tunnel: w357 -> [_ w391]
                tunnel: w351 -> [w366 w390]
                tunnel: w350 -> [w365 w389]
                tunnel: w349 -> [w364 w388]
                tunnel: w348 -> [w363 w387]
                frame False {
                  n149 = case shown="False" w369 {
                    tunnel: w370 -> [_ w385]
                    tunnel: w364 -> [_ w384]
                    tunnel: w366 -> [_ w383]
                    tunnel: w367 -> [w377 w381]
                    tunnel: [w377 w381] -> w368
                    tunnel: w363 -> [w379 _]
                    tunnel: w365 -> [w378 _]
                    tunnel: w371 -> [w375 _]
                    frame False {
                      n150 = call "Load_Zspec_param_data_SubVI.vi"("data\n\n 5"=w379, "Zspecparam.txt location"=w378) -> ("data"=w376:T1)  [unwired: 9 in]
                      n151 = Index Array(array=w376, index=w375) -> (element=w380:T9)
                      n152 = call "Update_ZSpec_Param_Data_SubVI.vi"("output cluster"=w380) -> ()  [unwired: 11 in]
                    }
                    frame True {
                      n153 = call "Load_STS_param_data_SubVI.vi"("data\n\n in"=w384, "STSparam.txt location"=w383) -> ("data\n\n out"=w382:T2)  [unwired: 9 in]
                      n154 = Index Array(array=w382, index=w385) -> (element=w386:T10)
                      n155 = call "Update_STS_Param_Data_SubVI.vi"("STSparameters"=w386) -> ()  [unwired: 11 in]
                    }
                  }
                  n156 = call "Update_Grid_Res_Drift_Correction_SubVI.vi"("Drift Correction Settings"=w373, "Boolean"=w372, "Experiment 6"=w368) -> ("Experiment 5"=w362:T8)  [unwired: 8 in]
                  n157 = local write "Experiment 5"(w362) -> ()
                  n158 = call "Start_Grid_SUbVI.vi"("Experiment 5"=w362) -> ("Drift Correction Settings"=w374:T11)  [unwired: 10 in]
                }
                frame True {
                  n159 = for {
                    N: w399 -> [_]
                    tunnel: w391 -> [w417] mode=indexing
                    tunnel: w398 -> [w416]
                    tunnel: w397 -> [w405]
                    tunnel: w396 -> [w406]
                    tunnel: w395 -> [w407]
                    shift-right: [w411] -> w394
                    shift-left: w393 -> [w415]
                    tunnel: w392 -> [w410]
                    tunnel: w390 -> [w404]
                    tunnel: w389 -> [w403]
                    tunnel: w388 -> [w402]
                    tunnel: w387 -> [w401]
                    i -> [w414]
                    n160 = call "Update_Repeat_Param_Value_SubVI.vi"("String"=w417, "Experiment 6"=w416) -> ("Experiment 5"=w409:T8)  [unwired: 9 in]
                    n161 = case shown="False" w405 {
                      tunnel: w406 -> [_ w428]
                      tunnel: w402 -> [_ w427]
                      tunnel: w404 -> [_ w426]
                      tunnel: w409 -> [w420 w425]
                      tunnel: [w420 w425] -> w408
                      tunnel: w401 -> [w422 _]
                      tunnel: w403 -> [w421 _]
                      tunnel: w407 -> [w418 _]
                      frame False {
                        n162 = call "Load_Zspec_param_data_SubVI.vi"("data\n\n 5"=w422, "Zspecparam.txt location"=w421) -> ("data"=w419:T1)  [unwired: 9 in]
                        n163 = Index Array(array=w419, index=w418) -> (element=w423:T9)
                        n164 = call "Update_ZSpec_Param_Data_SubVI.vi"("output cluster"=w423) -> ()  [unwired: 11 in]
                      }
                      frame True {
                        n165 = call "Load_STS_param_data_SubVI.vi"("data\n\n in"=w427, "STSparam.txt location"=w426) -> ("data\n\n out"=w424:T2)  [unwired: 9 in]
                        n166 = Index Array(array=w424, index=w428) -> (element=w429:T10)
                        n167 = call "Update_STS_Param_Data_SubVI.vi"("STSparameters"=w429) -> ()  [unwired: 11 in]
                      }
                    }
                    n168 = Equal To 0?(x=w414) -> (x = 0?=w413:bool)
                    n169 = And(x=w410, y=w413) -> (x .and. y?=w412:bool)
                    n170 = call "Update_Grid_Res_Drift_Correction_SubVI.vi"("Drift Correction Settings"=w415, "Boolean"=w412, "Experiment 6"=w408) -> ("Experiment 5"=w400:T8)  [unwired: 8 in]
                    n171 = local write "Experiment 5"(w400) -> ()
                    n172 = call "Start_Grid_SUbVI.vi"("Experiment 5"=w400) -> ("Drift Correction Settings"=w411:T11)  [unwired: 10 in]
                  }
                }
              }
              n173 = local write "size(s) 5"(w347) -> ()
            }
          }
        }
      }
      event "Update STS/Zspec Param List": Value Change {
        n174 = event-data() -> ()  [unwired: 1 in, 6 out]
        n175 = local read "STSparam.txt location"() -> (w436:path)
        n176 = local read "Zspecparam.txt location"() -> (w435:path)
        n177 = control-ref of="data\n\n 2"() -> (w434:refnum<vi>)
        n178 = call "Load_STS_param_options_SubVI.vi"("STSparam.txt location"=w436, "Array in"=w434) -> ("error out"=w437:errorcluster, "Array"=w431:string[])  [unwired: 8 in]
        n179 = control-ref of="data\n\n 5"() -> (w433:refnum<vi>)
        n180 = call "Load_Zspec_param_options_SubVI.vi"("error in (no error)"=w437, "Zspecparam.txt location"=w435, "Array in"=w433) -> ("Array"=w432:string[])  [unwired: 8 in]
        n181 = for {
          N: 5 -> [_]
          tunnel: w432 -> [w439]
          tunnel: w431 -> [w438]
          i -> [w440]
          n182 = case shown="2" w440 {
            tunnel: w439 -> [w442 w444 w446 w448 w450]
            tunnel: w438 -> [w441 w443 w445 w447 w449]
            frame 0, Default {
              n183 = property on="STS Param List #1" class="Ring (strict)"("Strings []"=w441) -> ()  [unwired: 2 in, 2 out]
              n184 = property on="ZSpec Param List #1" class="Ring (strict)"("Strings []"=w442) -> ()  [unwired: 2 in, 2 out]
            }
            frame 1 {
              n185 = property on="STS Param List #2" class="Ring (strict)"("Strings []"=w443) -> ()  [unwired: 2 in, 2 out]
              n186 = property on="ZSpec Param List  #2" class="Ring (strict)"("Strings []"=w444) -> ()  [unwired: 2 in, 2 out]
            }
            frame 2 {
              n187 = property on="STS Param List #3" class="Ring (strict)"("Strings []"=w445) -> ()  [unwired: 2 in, 2 out]
              n188 = property on="ZSpec Param List #3" class="Ring (strict)"("Strings []"=w446) -> ()  [unwired: 2 in, 2 out]
            }
            frame 3 {
              n189 = property on="STS Param List #4" class="Ring (strict)"("Strings []"=w447) -> ()  [unwired: 2 in, 2 out]
              n190 = property on="ZSpec Param List  #4" class="Ring (strict)"("Strings []"=w448) -> ()  [unwired: 2 in, 2 out]
            }
            frame 4 {
              n191 = property on="STS Param List #5" class="Ring (strict)"("Strings []"=w449) -> ()  [unwired: 2 in, 2 out]
              n192 = property on="ZSpec Param List #5" class="Ring (strict)"("Strings []"=w450) -> ()  [unwired: 2 in, 2 out]
            }
          }
        }
      }
      event "stop": Value Change {
        n193 = event-data() -> ()  [unwired: 1 in, 4 out]
      }
    }
    n194 = Wait (ms)(milliseconds to wait=u32 100) -> ()  [unwired: 1 out]
  }
